vi "AlliGator Decay Analysis Actions.vi"(0 "AlliGator Q Elements in":T6[](array[typedef]), 1 "VI in":refnum<vi>, 2 "Script in":bool, 5 "AlliGator IV DVR in":refnum<data-value>, 7 "AlliGator Q Event in":T7=enum."GUI:Idle", 9 "Data":variant, 11 "error in (no error)":errorcluster, 12 "AlliGator Ctrl Refnums":T8) -> (3 "Script off":bool, 4 "AlliGator Q Elements out":T6[](array[typedef]), 6 "AlliGator IV DVR out":refnum<data-value>, 10 "[Notebook Message]":T1[](array[typedef]) {"Message Style"."Font Size" min=6.0 step=1.0}, 15 "error out":errorcluster)   [LabVIEW 2021, in "AlliGator Action Engine.lvlib"]
doc: "Processes AlliGator decay-related actions."
uses:
  AlliGator Action Engine.lvlib
  Internal Variables/AlliGator Internal Variables v2.ctl
  <vilib>/vision/Image Controls.llb/IMAQ Image.ctl
  Internal Variables/AlliGator Gate Image Set.ctl
  Files/AlliGator FLI Dataset Type.ctl
  Files/AlliGator Data Series Type.ctl
  Dual-Channel Datasets/AlliGator Dataset Channel.ctl
  Settings/AlliGator Gate Arithmetic.ctl
  Source Image/AlliGator Displayed Image.ctl
  Image/Named ROI Description.ctl
  Phasor Graph/AlliGator Decay Metadata v3.ctl
  Decay Analysis/Decay Preprocessing/AlliGator Decay Background Subtraction Info.ctl
  Decay Analysis/Decay Preprocessing/AlliGator Baseline Subtraction Method.ctl
  Graphs/XY Graph/XY Graph Plot Shift Parameters.ctl
  Graphs/XY Graph/XY Graph Plot Shift Method.ctl
  Decay Analysis/Decay Preprocessing/AlliGator Decay Extrapolation Parameters.ctl
  Phasor/Calibration Phasor (m, phi).ctl
  Phasor/Phasor Reference Series.ctl
  Phasor/Phasor Calibration Map v2.ctl
  Phasor/Phasor (g, s).ctl
  Phasor Graph/AlliGator Raw Phasor Plot Data v5.ctl
  Phasor/Phasor Standard Deviation Options.ctl
  Phasor Plot/AlliGator Phasor Multi-Harmonic Data.ctl
  Phasor/Phasor Harmonic Data.ctl
  Decay Fit Parameter Map/AlliGator Decay Fit Options & Parameters v4.ctl
  Fits/IRF(X)PSED/Decay Fit Options v4.ctl
  Fits/Decay Convolution/Decay Model.ctl
  Fits/Residual Type.ctl
  Fits/IRF(X)PSED/Fit Weights Type v2.ctl
  Fits/Non-linear Fitting Method v2.ctl
  Fits/Fit Calculation Method.ctl
  Fits/Non-linear Fitting Algorithm.ctl
  Decay Analysis/Decay Fit/AlliGator Decay Fit Parameter Constraints 2.ctl
  Fits/IRF(X)PSED/Decay Fit Parameters In List.ctl
  Fits/IRF(X)PSED/MLE Baseline Offset Type.ctl
  Decay Analysis/Decay Preprocessing/AlliGator Decay Preprocessing Parameters.ctl
  Fits/IRF(X)PSED/Decay Fit Parameters & Derived Quantities List v2.ctl
  Fits/IRF(X)PSED/Decay Fit Result Constraint.ctl
  Decay Fit Parameter Map/AlliGator Parameter Maps Data.ctl
  AlliGator Q Event.ctl
  GUI/AlliGator Ctrl Refnums.ctl
  GUI/AlliGator Other Ctrl Refnums.ctl
  GUI/AlliGator State Indicator.ctl
  GUI/AlliGator Main Window Tabs.ctl
  GUI/AlliGator Phasor Plot Ctrl Refnums.ctl
  GUI/AlliGator Phasor Graph Ctrl Refnums.ctl
  Phasor/Phasor Calibration Type.ctl
  GUI/AlliGator Dataset Ctrl Refnums.ctl
  GUI/AlliGator Registered Events Ctrl Refnums.ctl
  GUI/AlliGator Image Histogram Control Refnums.ctl
  Histograms/Linear Histogram Options.ctl
  Histograms/Histogram Bin Option.ctl
  Histograms/Histogram Bin Position.ctl
  Decay Fit Parameter Map/AlliGator Decay Fit Map Control Refnums.ctl
  Parameter Map/AlliGator Parameter Map Control Refnums.ctl
  AlliGator Q Element.ctl
  Notebook/Notebook Message Object.ctl
  Rich Text Box/Text Formatting.ctl
  Rich Text Box/Text Colors.ctl
  Rich Text Box/Text Style.ctl
  Rich Text Box/Text Alignment.ctl
  Rich Text Box/Text Format List.ctl
  Graphs/LabVIEW Plot Interpolation.ctl
  Graphs/Plot Point Style.ctl
  <vilib>/Utility/miscctls.llb/LVPoint32TypeDef.ctl
  Alligator Elements Order in Action Stack.ctl
  AlliGator State Indicators List.ctl
  Settings/AlliGator Settings List.ctl
  Graphs/XY Graph/XY Graph Selected Plot Info+Flag.ctl
  Graphs/XY Graph/XY Graph Refnum.ctl
  Fits/Square Pulse/Square Pulse Options.ctl
  Fits/Square Pulse/Square Pulse Levels Type.ctl
  Graphs/XY Graph/XY Graph Selected Plot Info.ctl
  Variant/Variant to Data/Variant to I32.vi
  AlliGator Add Single Action to Stack.vi
  AlliGator Add Action Array to Stack.vi
  Variant/Variant to Data/Variant to U32.vi
  Variant/Variant to Data/Variant to DBL.vi
  GUI/GUI.lvlib
  Decay Analysis/IRF/AlliGator IRF.lvlib
  Variant/Variant to Data/Variant to Data.lvlib
  GUI/AlliGator GUI.lvlib
  Decay Analysis/Decay Fit/AlliGator Decay Fit.lvlib
  Graphs/XY Graph/XY Graph Add-Ons.lvlib
  Decay Analysis/Decay Processing/AlliGator Decay Processing.lvlib
  Settings/AlliGator Settings.lvlib
  Internal Variables/AlliGator Internal Variables.lvlib
  Fits/Fits.lvlib
  Decay Analysis/Decay Preprocessing/AlliGator Decay Preprocessing.lvlib
  Graphs/Graphs.lvlib
  Decay Analysis/Global Decay Fit/AlliGator Global Decay Fit.lvlib
  Sound/Sound.lvlib
  Fits/Abort Fit Global.vi
  Intensity Corrections/AlliGator Intensity Corrections.lvlib
  Strings/Strings.lvlib
  Notebook/Notebook.lvlib
  Phasor/Phasor.lvlib
  Image/Image.lvlib
  Phasor Graph/AlliGator Phasor Graph.lvlib
  Files/AlliGator Files.lvlib
  Phasor Plot/AlliGator Phasor Plot.lvlib
  Source Image/AlliGator Source Image.lvlib
  Decay Fit Parameter Map/AlliGator Decay Fit Parameter Map.lvlib
  Rich Text Box/Rich Text Box.lvlib
  Dual-Channel Datasets/AlliGator Dual-Channel Datasets.lvlib
  Histograms/Histogram Window.lvlib
  Parameter Map/AlliGator Parameter Map.lvlib
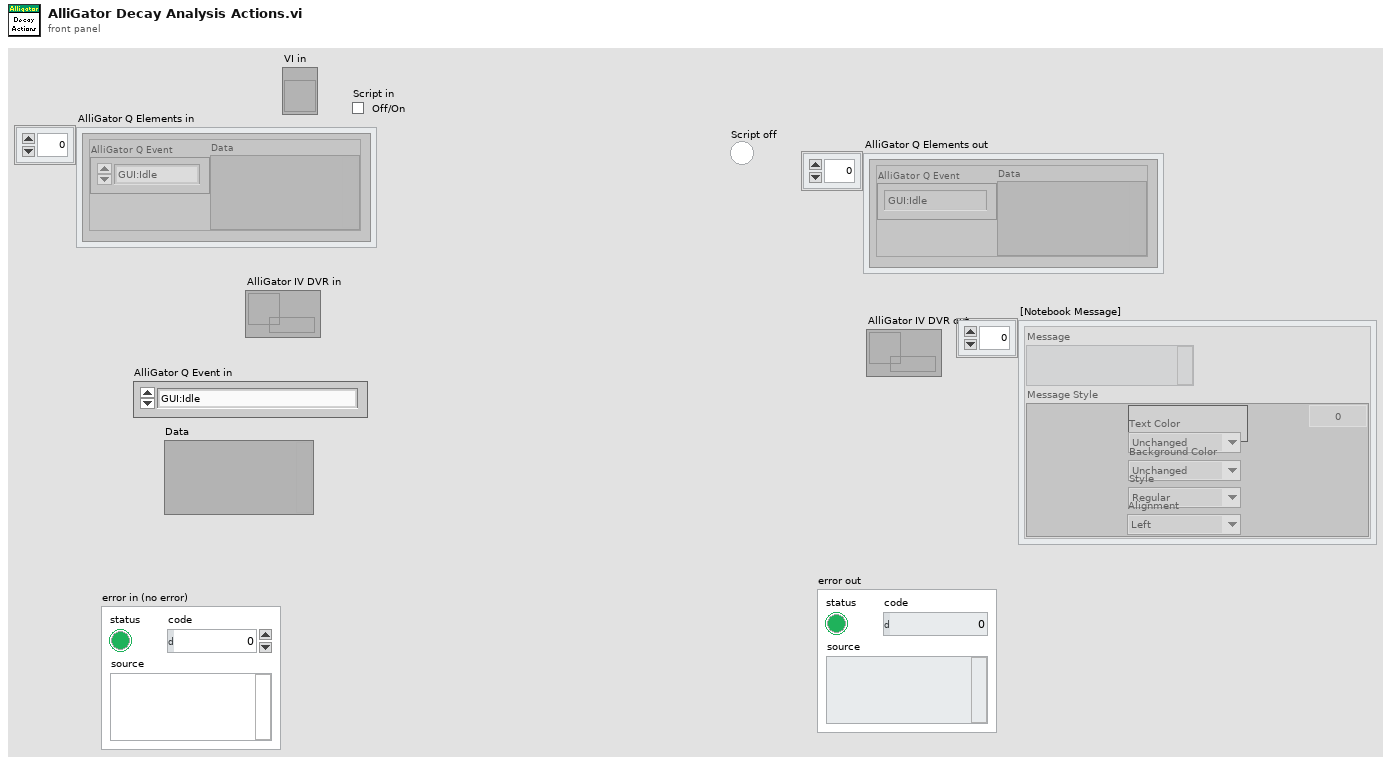
[diagram p1: front panel]
types:
  T1 = typedef "Notebook.lvlib/Notebook Message Object.ctl" = cluster{"Message":string, "Message Style":T2}
  T2 = typedef "Rich Text Box.lvlib/Text Formatting.ctl" = cluster{"Font":string, "Text Color":T3, "Background Color":T3, "Style":T4, "Font Size":dbl, "Alignment":T5}
  T3 = typedef "Rich Text Box.lvlib/Text Colors.ctl" = enum16{"Unchanged", "Black", "Blue", "Cyan", "Maroon", "Gray", "Violet", "Green", "Light Green", "Orange", "Yellow", "Magenta", "Red", "White"}
  T4 = typedef "Rich Text Box.lvlib/Text Style.ctl" = enum16{"Regular", "Bold", "Italic", "Underline", "Strikeout"}
  T5 = typedef "Rich Text Box.lvlib/Text Alignment.ctl" = enum16{"Left", "Right", "Center"}
  T6 = typedef "AlliGator Action Engine.lvlib/AlliGator Q Element.ctl" = cluster{"AlliGator Q Event":T7, "Data":variant}
  T7 = typedef "AlliGator Action Engine.lvlib/AlliGator Q Event.ctl" = enum16{"---- Files ----", "Files:Set Batch Export Files To Save", "Files:Set Dataset Loading & Pre-processing Options", "Files:Check #Frames in Dataset", "Files:Increment Frame Index", "Files:Open Mask Image", "Files:Open White Light Image", "Files:Open Single Dataset", "Files:New Folder of Folders Selected", "Files:Load File (all Types)_Scriptable", "Files:Move Flattened Series to Folders Series", "Files:Select Folder", "Files:Load FLI Dataset", "Files:Load Swiss SPAD 1 Dataset", "Files:Load Swiss SPAD 2 Dataset", "Files:Load .sdt FLI Dataset", "Files:Load .ptu FLI Dataset", "Files:Load .bin FLI Dataset", "Files:Load Single Gate Image Folder", "Files:Load I/m/phi Dataset (deprecated)", "Files:Load Single Image", "Files:Subtract Background File", "Files:Export FLI Dataset", "Files:Load HDF5 FLI Dataset", "Files:Set Destination File Path", "Files:Save Mask Image", "Files:Batch Conversion", "Files:New Folder Selected", "Files:Close FLI Dataset", "Files:Close FLI Dataset Series", "Files:Close White Light Image", "Files:Close Mask Image", "---- FLI Dataset ----", "FLI Dataset:Channel Arithmetic", "FLI Dataset:Export Average Lifetime Map as ASCII", "FLI Dataset:Export User-Defined Quantity Map as ASCII", "FLI Dataset:Python Function FLI Dataset Event", "FLI Dataset:ROI Analysis", "FLI Dataset:Tilted Logistic Square Gated IRF Characteristics Map", "FLI Dataset:Logistic Square Gated IRF Characteristics Map", "FLI Dataset:Square Gated IRF Characteristics Map", "FLI Dataset:Multi-ROI Single-Pixel Phasor Analysis", "FLI Dataset:Multi-ROI Single-Pixel NLSF Analysis", "FLI Dataset:All ROIs IRF Extraction", "FLI Dataset:All ROIs Decay Fit Non-Interactive (Fast + Individual IRF)", "FLI Dataset:All ROIs Phasor Analysis", "FLI Dataset:All ROIs Decay Fit", "FLI Dataset:Fluorescence Decay Statistics", "FLI Dataset:Update Decay Statistics Graph", "FLI Dataset:Get Decay from ROI", "FLI Dataset:All ROIs Average Lifetimes", "FLI Dataset:Save/Load Local IRFs", "FLI Dataset:Clear Local IRFs", "FLI Dataset:Phasor Calibration Maps (# Gates Series) Script", "FLI Dataset:Calibrated Phasor Map Series", "---- FLI Dataset Series ----", "FLI Dataset Series:Sum All Datasets in Series", "FLI Dataset Series:Add Dataset to Accumulated Dataset", "FLI Dataset Series:Display Accumulated Dataset", "FLI Dataset Series:Clear Dataset Series Sum", "FLI Dataset Series:Time-Series Analysis (NLSF)", "FLI Dataset Series:Time-Series Analysis (Phasor)", "---- Image ----", "Image:Update Image Profile Plots", "Image:Image Histogram Cursor Move", "Image:Image Histogram", "Image:Image Contrast", "Image:Set Image Histogram Cursor Move Flag", "Image:Clear Image Overlay", "Image:Use ROI as Search Area", "Image:Set ROI Diameter", "Image:Save Image Data as TIFF", "Image:Save Displayed Image with Overlay", "Image:Save Image Overlay Only", "Image:Save Image as Hot Pixel Mask", "Image:Change Source Image Color Palette", "Image:Copy Image to Clipboard", "Image:Source Image ROI Selection", "Image:Delete All ROIs", "Image:Delete All Unselected ROIs", "Image:Delete ROI", "Image:Merge All ROIs", "Image:Store ROI", "Image:Source Image ROI Storage", "Image:Export ROI Description to Notebook", "Image:Save ROI", "Image:Load ROI", "Image:Paste ROI Definition", "Image:Clear ROI", "Image:Identify ROIs in Mask Image", "Image:Create Complementary ROI", "Image:Create Contour ROI", "Image:Create ROI(s) from Pixels with Peak above Min_Scriptable", "Image:Create ROI(s) from Pixels with Intensity above Min_Scriptable", "Image:Compute ROI Statistics", "Image:Delete ROI(s) based on ROI Characteristics", "Image:Create ROI Grid", "Image:ROI to Individual Pixel ROIs", "Image:Python Function Source Image Event", "Image:Show Phasor Calibration Map ROI Centers", "Image:Convert ROI to Mask Image", "Image:Mouse Move", "Image:Mouse Up", "Image:Set Source Image Mouse Move Flag", "Image:Add Scale Bar Overlay", "Image:Delete Existing ROIs Option", "Image:Overlay ROI Median", "Image:Check Current ROI", "Image:Update True Pixel Value", "---- Decay ----", "Decay:Clear IRF/Reference Plot", "Decay:Add Decay to Graph", "Decay:Smoothen Plot", "Decay:Smoothen Plot Tail", "Decay:Average Selected Plots", "Decay:Extract IRF", "Decay:Optimal IRF Extraction", "Decay:Threshold IRF", "Decay:Fit to Model IRF", "Decay:Fit IRF to Square Gate", "Decay:Fit IRF to Logistic Square Gate", "Decay:Fit IRF to Tilted Logistic Square Gate", "Decay:Create Bounding Cursors Set", "Decay:Export Bounding Cursors Definition to Notebook", "Decay:Denoise Plot", "Decay:Compute Cumulative Function", "Decay:Use as Reference Decay", "Decay:Show Reference Decay/IRF", "Decay:Extrapolate Decay", "Decay:Create Head & Tail Bounding Cursors", "Decay:Store Cursor-defined Head & Tail Fractions", "Decay:Rebin Plot", "Decay:1-Normalize Decay", "Decay:[0-1]-Normalize Plot", "Decay:Straighten Decay", "Decay:Shift Decay", "Decay:Fold Decay", "Decay:Fit Decay", "Decay:Global Fit of Selected Decays", "Decay:Post Global Fit Script", "Decay:Add Global Fit Parameters to Graph", "Decay:Add Decay Parameter(s) to Plot (Graph)", "Decay:Export Decay to Phasor Graph", "Decay:Compute Average Lifetime", "Decay:Plot Convolution", "Decay:Graph Tip Strip Update", "---- Decay Statistics ----", "Decay Statistics:Tip Strip Update", "---- Intensity Time Trace ----", "Intensity Time Trace:Use File Timestamp", "Intensity Time Trace:Load Intensity Corrections File", "Intensity Time Trace:Clear Intensity Corrections File", "Intensity Time Trace:Tip Strip Update", "---- Phasor Plot ----", "Phasor Plot:Build Phasor Plot", "Phasor Plot:Change Phasor Plot Color Palette", "Phasor Plot:Adjust Phasor Plot Display Range", "Phasor Plot:Highlight Image ROI in Phasor Plot", "Phasor Plot:Save Phasor Plot Image with Overlay", "Phasor Plot:Export Complex Phasor Map", "Phasor Plot:Export Phasor Ratio Map", "Phasor Plot:Export Average Lifetime Map", "Phasor Plot:Compute Phase Lifetime Histogram", "Phasor Plot:Compute Phasor Ratio Histogram", "Phasor Plot:Compute Phase Lifetime vs Intensity Scatter Plot", "Phasor Plot:Weber 2-Component Decomposition", "Phasor Plot:Update Phasor Color Map Vertices", "Phasor Plot:Clear Phasor Overlay", "Phasor Plot:Use Segment Extremities as References", "Phasor Plot:Use UC/Segment Intersections as References", "Phasor Plot:Use UC/Principal Axis Intersections as References", "Phasor Plot:Use UC/Linear Fit Intersections as References", "Phasor Plot:Update Phasor Plot Reference", "Phasor Plot:Show Local Phasor Info in Phasor Plot", "Phasor Plot:Update Phasor Plot State", "Phasor Plot:Phasor Plot ROI Storage", "Phasor Plot:Phasor Plot ROI Selection", "Phasor Plot:Python Function Phasor Plot Event", "Phasor Plot:Overlay Phasor ROI, Ratio or Map in Source Image", "Phasor Plot:Compute Decay of Selected Phasors", "Phasor Plot:Phasor at Image Pixel", "Phasor Plot:Mouse Move", "Phasor Plot:Mouse Up", "Phasor Plot:Display Range Mouse Move", "Phasor Plot:Set Mouse Move Flag", "Phasor Plot:Update True Phasor Plot Value", "---- Phasor Graph ----", "Phasor Graph:Get Phasor Value", "Phasor Graph:Create New Phasor Plot Dialog", "Phasor Graph:Update Last Phasor Value", "Phasor Graph:Update Phasor (m, phi)", "Phasor Graph:Remove Single Phasor from Plot", "Phasor Graph:Add Single Phasor to Plot", "Phasor Graph:Remove Phasor Plot", "Phasor Graph:Remove Selected Phasor Plots", "Phasor Graph:Clear Phasor Data", "Phasor Graph:Clear Phasor Graph", "Phasor Graph:Cursor Move", "Phasor Graph:Draw Cursor Connecting Line", "Phasor Graph:Clear Cursor Connecting Line", "Phasor Graph:Find UC Intersection", "Phasor Graph:Use UC/Cursor-Defined Line Intersections", "Phasor Graph:Use Selected Plots Fitted Line/UC Intersections", "Phasor Graph:Use Selected Plots Principal Axis/UC Intersections", "Phasor Graph:Show Single Phasor", "Phasor Graph:Save Single Phasor Plot", "Phasor Graph:Save All Phasor Plots", "Phasor Graph:Load Phasor Plot(s)", "Phasor Graph:Phasor Multiplication", "Phasor Graph:Compute Average Phasor", "Phasor Graph:Compute Multiple Average Phasors (Selected Plots)", "Phasor Graph:Export Single Phasor Plot Phase Lifetimes", "Phasor Graph:Parameter 2 vs Parameter 1 Scatter Plot", "Phasor Graph:Use Cursor n Location", "Phasor Graph:Set Reference n to Current Phase Lifetime Value", "Phasor Graph:Set Reference n to Lifetime Value", "Phasor Graph:Set Cursor n Location", "Phasor Graph:Save Phasor Graph Image", "Phasor Graph:Update SEPL Plot", "Phasor Graph:Export Single Phasor Plot Data", "Phasor Graph:Export Selected Phasor Plots Data", "Phasor Graph:Python Function Phasor Graph Event", "Phasor Graph:Tip Strip Update", "---- Calibration ----", "Calibration:Set Calibration Type", "Calibration:Load/Save Phasor Calibration", "Calibration:Load/Save Phasor Calibration Series", "Calibration:Load/Save Phasor Calibration Map", "Calibration:Use as Calibration", "Calibration:Compute Optimal Calibration from Phasor References", "Calibration:Clear Phasor Calibration", "Calibration:Single Phasor Calibration Information", "Calibration:Use as Calibration Series", "Calibration:Use as Calibration Map", "Calibration:Clear Calibration Series", "Calibration:Phasor Calibration Series Information", "Calibration:Clear Calibration Map", "Calibration:Phasor Calibration Map Information", "Calibration:Apply Phasor Calibration", "Calibration:Update Single Plot Calibration", "Calibration:Update Multiple Plots Calibration", "Calibration:Clear Single Plot Calibration", "Calibration:Clear All Plots Calibrations", "Calibration:Clear Plot(s) Calibration(s)?", "---- Phasor Ratio ----", "Phasor Ratio:Clear Reference n", "Phasor Ratio:Toggle Selected Plot(s)  Lock to Reference 1", "Phasor Ratio:Use as Reference n", "Phasor Ratio:Send Reference n to Notebook", "Phasor Ratio:Toggle Selected Plot(s)  Lock to Reference 2", "Phasor Ratio:Compute Phasor Ratio at Mouse Location", "Phasor Ratio:Compute Phasor Plot's Average Phasor Ratio", "Phasor Ratio:Compute Time-Series Phasor Ratios", "Phasor Ratio:Fit Line to Phasor Ratio Plot", "Phasor Ratio:Save References", "Phasor Ratio:Load References", "Phasor Ratio:Update Phasor Reference 1", "Phasor Ratio:Update Phasor Reference 2", "Phasor Ratio:Move Cursor n to Reference n", "Phasor Ratio:Use as Phasor Reference 1 Lifetime", "Phasor Ratio:Use as Phasor Reference 2 Lifetime", "Phasor Ratio:Export Phasor Ratio Map as ASCII", "Phasor Ratio:Tip Strip Update", "---- Lifetime & Other Parameters Graph ----", "Lifetime:Compute Sliced Mean, SDV and CV Plots", "Lifetime:Plot Decay Shifts", "Lifetime:Plot Histogram", "---- Decay Fit Parameter Map ----", "Decay Fit Parameter Map:Export ROI NLSF Data as ASCII", "Decay Fit Parameter Map:Set Decay Fit Parameter Map Selection", "Decay Fit Parameter Map:Build Decay Fit Parameter Map", "Decay Fit Parameter Map:Change Decay Fit Parameter Map Color Palette", "Decay Fit Parameter Map:Export Decay Fit Parameter Map Data as ASCII", "Decay Fit Parameter Map:Export All Decay Fit Parameter Maps Data as ASCII", "Decay Fit Parameter Map:Selected Parameter Scatterplot", "Decay Fit Parameter Map:Parameter 2 vs Parameter 1 Scatterplot", "Decay Fit Parameter Map:Save Decay Fit Parameter Map Image", "Decay Fit Parameter Map:Save-Load IRFs & Fit Data", "Decay Fit Parameter Map:Update Local Decay Plots", "Decay Fit Parameter Map:Python Function Decay Fit Parameters Map Event", "Decay Fit Parameter Map:Overlay Decay Fit Parameter Map in Source Image", "Decay Fit Parameter Map:Selected Parameter vs Intensity Scatterplot", "Decay Fit Parameter Map:Mouse Up", "Decay Fit Parameter Map:Mouse Move", "Decay Fit Parameter Map:Display Range Mouse Move", "Decay Fit Parameter Map:Change Map Resolution", "Decay Fit Parameter Map:Variance Significance Maps", "Decay Fit Parameter Map:Fit Result Constraints Window", "---- Parameter Map ----", "Parameter Map:Export ROI Parameters Data as ASCII", "Parameter Map:Add Parameter Map Set", "Parameter Map:Delete Parameter Map Set", "Parameter Map:Update Parameter List", "Parameter Map:Build Parameter Map", "Parameter Map:Change Parameter Map Color Palette", "Parameter Map:Export Parameter Map Data as ASCII", "Parameter Map:Export All Parameter Maps Data as ASCII", "Parameter Map:Selected Parameter Scatterplot", "Parameter Map:Parameter 2 vs Parameter 1 Scatterplot", "Parameter Map:Selected Parameter vs Intensity Scatterplot", "Parameter Map:Save Parameter Map Image", "Parameter Map:Save-Load IRFs & Parameter Maps (TODO)", "Parameter Map:Set Parameter Map Selection", "Parameter Map:Python Function Parameter Map Event", "Parameter Map:Overlay Parameter Map in Source Image", "Parameter Map:Update Local Decay Plots", "Parameter Map:Mouse Up", "Parameter Map:Mouse Move", "Parameter Map:Display Range Mouse Move", "---- Generic Graph ----", "Generic Graph:Generic XY Graph Event", "Generic Graph:Python Function XY Graph Event", "Generic Graph:New Plot", "Generic Graph:Save Plot", "Generic Graph:XY Plot Histogram", "Generic Graph:Set XY Graph Plot Name", "Generic Graph:Set Last Cursor Style", "Generic Graph:Tip Strip Update", "---- GUI ----", "GUI:Start Script", "GUI:Type of Displayed Image Changed", "GUI:Gate Image Slide Changed", "GUI:Show Busy Icon", "GUI:Show Busy Icon & Abort Button", "GUI:Hide Busy Icon", "GUI:Hide Busy Icon & Abort Button", "GUI:Abort", "GUI:End Script", "GUI:Start Timing", "GUI:End Timing", "GUI:Set State Indicator", "GUI:Send Parameters JSON Strings to Clipboard", "GUI:Set Gate Step", "GUI:Idle", "GUI:Initialization", "GUI:Quit", "GUI:Increment Dataset Index", "GUI:Set Dataset Index to -1", "GUI:Time Series Slider Moved", "GUI:Time Series Slider Changed", "GUI:Toggle Playback or Loop", "GUI:Playback Script", "GUI:Set Phasor Frequency", "GUI:Open Window", "GUI:Start Test Script", "GUI:End Test Script", "GUI:Set Verbose Mode", "GUI:Set Verbose Settings Mode", "DEBUG"}
  T8 = typedef "AlliGator GUI.lvlib/AlliGator Ctrl Refnums.ctl" = cluster{"Other AlliGator Ctrl Refnums":T9, "Phasor Plot Ctrl Refnums":T10, "Phasor Graph Ctrl Refnums":T11, "Dataset Control Refnums":T12, "Registered Events Ctrl Refnums":T13, "Image Histogram Ctrl Refnums":T14, "Decay Fit Map Ctrl Refnums":T15, "Parameter Map Ctrl Refnums":T16}
  T9 = typedef "AlliGator GUI.lvlib/AlliGator Other Ctrl Refnums.ctl" = cluster{"State Indicators":refnum<vi>, " Progress Bar":refnum<vi>, "Decay Graph Active":refnum<vi>, "Decay Statistics Bin":refnum<vi>, "Time Step":refnum<vi>, "Use File Timestamp":refnum<vi>, "Tab Control":refnum<vi>, "CPU":refnum<vi>, "Abort Fit":refnum<vi>, "Dataset File/Folder Path":refnum<vi>, "Abort ROI Creation":refnum<vi>, "Event LED":refnum<vi>, "Dataset File/Folder Path 2":refnum<vi>, "Dataset File/Folder Path 3":refnum<vi>, "Dataset File/Folder Path 4":refnum<vi>, "Dataset File/Folder Path 5":refnum<vi>, "Dataset File/Folder Path 6":refnum<vi>, "Dataset File/Folder Path 7":refnum<vi>, "Dataset File/Folder Path 8":refnum<vi>, "Dataset File/Folder Path 9":refnum<vi>, "Dataset File/Folder Path 10":refnum<vi>, "Dataset File/Folder Path 11":refnum<vi>}
  T10 = typedef "AlliGator GUI.lvlib/AlliGator Phasor Plot Ctrl Refnums.ctl" = cluster{"Phasor Ratio":refnum<vi>, "Modulus Lifetime":refnum<vi>, "Phasor at cursor (m, phi)":refnum<vi>, "Phase Lifetime":refnum<vi>, "Phasor at cursor (g, s)":refnum<vi>, "Phasor Plor Average Lifetime":refnum<vi>, "Phasor Plot Active":refnum<vi>, "Save Phasor Plot":refnum<vi>, "Image Overlay Color":refnum<vi>, "Phasor Plot Color Scale":refnum<vi>, "Reference 1 Button":refnum<vi>, "Reference 2 Button":refnum<vi>, "True Phasor Plot Value":refnum<vi>}
  T11 = typedef "AlliGator GUI.lvlib/AlliGator Phasor Graph Ctrl Refnums.ctl" = cluster{"Phasor Ratio":refnum<vi>, "Modulus Lifetime":refnum<vi>, "Phasor at cursor (m, phi)":refnum<vi>, "Phase Lifetime":refnum<vi>, "Phasor at cursor (g, s)":refnum<vi>, "Phasor Graph Average Lifetime":refnum<vi>, "Phasor Graph Active":refnum<vi>, "Save Phasor Graph":refnum<vi>, "Phasor Frame Slide":refnum<vi>, "Single Step Phasor":refnum<vi>, "Calibration Type":refnum<vi>, "Show Line":refnum<vi>, "Phase Lifetime 1":refnum<vi>, "Phase Lifetime 2":refnum<vi>, "Phasor Graph Frequency":refnum<vi>, "Phasor Reference 1 Control":refnum<vi>, "Phasor Reference 2 Control":refnum<vi>, "Calibration Lifetime":refnum<vi>, "Phase Lifetime SDV":refnum<vi>, "Average Lifetime SDV":refnum<vi>, "Phasor Ratio SDV":refnum<vi>, "Modulus Lifetime SDV":refnum<vi>}
  T12 = typedef "AlliGator GUI.lvlib/AlliGator Dataset Ctrl Refnums.ctl" = cluster{"Current Data":refnum<vi>, "Gate Image Slide":refnum<vi>, "Time Point Slide":refnum<vi>, "Current Time Stamp":refnum<vi>, "Save Image":refnum<vi>, "Displayed Image":refnum<vi>, "Overlay Mode":refnum<vi>, "Phasor Overlay Color":refnum<vi>, "Image Color Scale":refnum<vi>, "Use ROI as Search Area":refnum<vi>, "Source Image ROI Color":refnum<vi>, "True Pixel Value":refnum<vi>}
  T13 = typedef "AlliGator GUI.lvlib/AlliGator Registered Events Ctrl Refnums.ctl" = cluster{"Time Point Slider":refnum<vi>, "Phasor Plot Display Range":refnum<vi>, "Decay Graph":refnum<vi>, "Decay Statistics Graph":refnum<vi>, "Intensity Time Trace":refnum<vi>, "Phasor Graph":refnum<vi>, "Phasor Ratio Graph":refnum<vi>, "Lifetime Graph":refnum<vi>, "Phasor Plot Display":refnum<vi>, "Source Image Display":refnum<vi>, "Decay Fit Parameter Map Display Range":refnum<vi>, "Decay Fit Parameter Map Display":refnum<vi>, "Parameter Map Display Range":refnum<vi>, "Parameter Map Display":refnum<vi>, "Phasor Plot Display Range":refnum<vi>}
  T14 = typedef "AlliGator GUI.lvlib/AlliGator Image Histogram Control Refnums.ctl" = cluster{"Image Histogram":refnum<vi>, "Image Histogram Options":refnum<vi>, "Image Histogram Active":refnum<vi>, "Image Histogram Upper Percentile":refnum<vi>, "Image Histogram Lower Percentile":refnum<vi>, "Auto-Adjust Contrast":refnum<vi>}
  T15 = typedef "AlliGator Decay Fit Parameter Map.lvlib/AlliGator Decay Fit Map Control Refnums.ctl" = cluster{"Decay Fit Parameter Map Color Scale":refnum<vi>, "Decay Fit Parameter":refnum<vi>, "Max Parameter":refnum<vi>, "Min Parameter":refnum<vi>, "Decay Fit Parameter Map Display":refnum<vi>, "Decay Fit Parameter Map Display Range":refnum<vi>, "Decay Parameter Map X":refnum<vi>, "Decay Parameter Map Y":refnum<vi>, "Decay Parameter Map Value":refnum<vi>}
  T16 = typedef "AlliGator Parameter Map.lvlib/AlliGator Parameter Map Control Refnums.ctl" = cluster{"Parameter Map Color Scale":refnum<vi>, "Map Parameter":refnum<vi>, "Max Parameter":refnum<vi>, "Min Parameter":refnum<vi>, "Parameter Map Display":refnum<vi>, "Parameter Map Display Range":refnum<vi>, "Parameter Map Set":refnum<vi>, "Parameter Map X":refnum<vi>, "Parameter Map Y":refnum<vi>, "Parameter Map Value":refnum<vi>}
  T17 = typedef "Notebook.lvlib/Text Format List.ctl" = enum16{"Message", "Result", "Error", "Setting", "Verbose", "Warning"}
  T18 = typedef "Graphs.lvlib/Plot Point Style.ctl" = enum16{"not defined", "None", "Empty Circle", "Filled Circle", "Thick Circle", "Dotted Circle", "Empty Square", "Filled Square", "Thick Square", "Dotted Square", "Small Filled Square", "Dot", "Cross", "Tiny Cross", "Large X", "Small x", "Diamond", "Small Empty Square"}
  T19 = typedef "Graphs.lvlib/LabVIEW Plot Interpolation.ctl" = enum16{"Point (.)", "Stepwise Right (--.)", "Line + Point (\\. /)", "Stepwise Left (.--)", "Stepwise Centered (-.-)", "Stepwise Vertical (|.|)", "Line (-)", "Use Previous Plot's Style"}
  T20 = typedef "AlliGator Action Engine.lvlib/Alligator Elements Order in Action Stack.ctl" = enum16{"Enqueue 2 AFTER 1", "Enqueue 2 BEFORE 1"}
  T21 = typedef "AlliGator Action Engine.lvlib/AlliGator State Indicators List.ctl" = enum16{"Phasor Calibration Defined", "Phasor Calibration Series Defined", "Phasor Calibration Map Defined", "Phasor Reference 1 Defined", "Phasor Reference 2 Defined", "Lifetime Reference 1 Defined", "Lifetime Reference 2 Defined", "Phasor Calibration Used", "Phasor Calibration Series Used", "Phasor Calibration Map Used", "Dataset Update Needed", "Phasor Plot Update Needed", "Reference/IRF Defined", "Individual IRFs Defined"}
  T22 = typedef "AlliGator Settings.lvlib/AlliGator Settings List.ctl" = enum16{"GUI:Visible Settings Tab", "GUI:Last Run Version", "Source Image:Use Image Histogram for Contrast", "Source Image:Low Count Pixels Rejection Options", "Source Image:High Count Pixels Rejection Options", "Source Image:Use Image Brightness", "Source Image:Blend Overlay with Image Background", "Source Image:Use Fixed ROI Diameter", "Source Image:ROI Diameter", "Source Image:ROI Center Color", "Source Image:Peak Threshold", "Source Image:Intensity Threshold", "Source Image:Image Binning Options", "Source Image:Image Smoothing Options", "Source Image:Image Histogram Active", "Source Image:Invert Binary Mask", "Source Image:Hot Pixel Removal", "Source Image:Overlay Analyzed ROI Center", "Source Image:Auto-Adjust Contrast", "Source Image:Histogram Lower Percentile", "Source Image:Histogram Upper Percentile", "Source Image:Save Source Image", "Source Image:Scale Bar Options", "Source Image:Image Resolution (Pixel Size)", "Source Image:Flatfield Correction", "Source Image:Show Dead Left Columns Correction", "Source Image:Dead Left Columns Correction", "Source Image:Image Pre-Processing Operations Order", "Source Image:Overlay ROI Median", "Source Image:Median Overlay Color", "Data Information:Gate Width", "Data Information:Nanotime Gate Separation", "Data Information:Macrotime Gate Separation", "Data Information:Gate Step", "Data Information:# Gates", "Data Information:Gate Image Exposure", "Data Information:Gate Image Integration", "Data Information:Gates to Skip", "Data Information:Gates to Keep", "Data Information:Define Gates to", "Data Information:Channel Name", "Data Information:Available Channel Names", "Data Information:Channel Arithmetic", "Data Information:Background File Subtraction", "Data Information:Background File", "Data Information:Background Scaling Factor", "Data Information:Background Pile-up Correction", "Data Information:Background Pixel Well Capacity", "Data Information:Laser Period", "Data Information:SYNC Period", "Data Information:Pile-up Correction", "Data Information:Pixel Well Capacity", "Data Information:Dataset Scaling Factor", "Fluorescence Decay_Decay Pre-Processing:Reverse Gates", "Fluorescence Decay_Decay Pre-Processing:Verbose Decay Pre-Processing", "Fluorescence Decay_Decay Pre-Processing:Use Decay Pre-Processing", "Fluorescence Decay_Decay Pre-Processing:Background Subtraction", "Fluorescence Decay_Decay Pre-Processing:Background Definition Range", "Fluorescence Decay_Decay Pre-Processing:Baseline Subtraction Method", "Fluorescence Decay_Decay Pre-Processing:Decay Pre-Processing Operations Order", "Fluorescence Decay_Decay Pre-Processing:Smoothing Parameter", "Fluorescence Decay_Decay Pre-Processing:Shift Decay", "Fluorescence Decay_Decay Pre-Processing:Decay Shift Parameters", "Fluorescence Decay_Decay Pre-Processing:Fold Decay", "Fluorescence Decay_Decay Pre-Processing:# Folds", "Fluorescence Decay_Decay Pre-Processing:1-Normalize Decay", "Fluorescence Decay_Decay Pre-Processing:[0-1]-Normalize Decay", "Fluorescence Decay_Decay Pre-Processing:Smoothen Decay", "Fluorescence Decay_Decay Pre-Processing:Extrapolate Decay", "Fluorescence Decay_Decay Pre-Processing:Use Periodicity", "Fluorescence Decay_Decay Pre-Processing:Use Cursors", "Fluorescence Decay_Decay Pre-Processing:Tail Fraction", "Fluorescence Decay_Decay Pre-Processing:Head Fraction", "Fluorescence Decay_Decay Pre-Processing:Additional Points", "Fluorescence Decay_Decay Pre-Processing:Straighten Decay", "Fluorescence Decay_Decay Pre-Processing:Constant Background", "Fluorescence Decay_Decay Pre-Processing:Pixel-Normalize Decay", "Fluorescence Decay_Advanced Analysis:Extract IRF instead of Decay", "Fluorescence Decay_Advanced Analysis:IRF Extraction Options", "Fluorescence Decay_Advanced Analysis:IRF Optimization Options", "Fluorescence Decay_Advanced Analysis:Square Pulse Options", "Fluorescence Decay_Advanced Analysis:IRF Order", "Fluorescence Decay_Advanced Analysis:IRF Time Constants", "Fluorescence Decay_Advanced Analysis:Wavelet Analysis Options", "Fluorescence Decay_Advanced Analysis:Average Lifetime Options", "Fluorescence Decay_Fit Options:Fit Options", "Fluorescence Decay_Fit Options:Use Legacy Fitting Approach", "Fluorescence Decay_Fit Options:Use Data Information Laser Period", "Fluorescence Decay_Fit Parameters:Displayed Fit Parameters", "Fluorescence Decay_Fit Parameters:Fit Parameter Constraints", "Fluorescence Decay_Fit Parameters:Export Tabulated Results", "Fluorescence Decay_Fit Parameters:MLE Baseline Offset Type", "Fluorescence Decay_Fit Parameters:MLE Baseline Offset", "Fluorescence Decay_Fit Parameters:Guess Parameter Names", "Fluorescence Decay_Fit Parameters:Guess Parameter Values", "Fluorescence Decay_Fit Parameters:Guess Parameters Options", "Fluorescence Decay_Fit Parameters:Optimal Offset Selection Criterion", "Fluorescence Decay_Styles:Show Last Decay Only", "Fluorescence Decay_Styles:Decay Graph Color Array", "Fluorescence Decay:Decay Graph Active", "Fluorescence Decay Statistics:Min Peak Value", "Fluorescence Decay Statistics:Reject Low Decay Peak Pixels", "Fluorescence Decay Statistics:Reject High Decay Peak Pixels", "Fluorescence Decay Statistics:Max Peak Value", "Time Traces:Use File Timestamp", "Time Traces:Time Step", "Time Traces:Use Intensity Correction File", "Time Traces:Intensity Correction File", "Phasor Plot:Phasor Plot Smoothing Options", "Phasor Plot:Phasor Plot Size", "Phasor Plot:Phasor Plot Graphics Options", "Phasor Plot:Cumulative Phasor Plot", "Phasor Plot:Use Phasor Brightness", "Phasor Plot:Blend Overlay with Phasor Background", "Phasor Plot:Save Phasor Plot", "Phasor Plot:Show References", "Phasor Plot:Phasor Ratio Decay Range", "Phasor Plot:Exponential Fading", "Phasor Plot:Phasor Ratio Reference Colors", "Phasor Plot:Reference Radius", "Phasor Plot:Show Color Map Vertices", "Phasor Plot:Phasor Plot Active", "Phasor Plot:Phasor Ratio Color Map Type", "Phasor Plot:Phasor Ratio Color Map", "Phasor Plot:Phasor Ratio Display Range", "Phasor Plot:Selected Image ROI(s)", "Phasor Plot:All Image ROIs", "Phasor Plot:Selected Phasor Plot ROI(s)", "Phasor Plot:All Phasor Plot ROIs", "Phasor Plot:Phasor Ratio Color-Coded Quantity", "Phasor Plot:Store Phasor Harmonics", "Phasor Plot:Draw Reference Segment", "Phasor Plot:User-Defined Quantity", "Phasor Plot:Color Scale High Color", "Phasor Plot:Color Scale Low Color", "Phasor Plot:Intensity-weighted Phasor Plot", "Phasor Graph:Phasor Frequency", "Phasor Graph:Phasor Ratio Type", "Phasor Graph:Pixel-level Phasor Computation", "Phasor Graph:Save Phasor Graph", "Phasor Graph:Phasor Graph Active", "Phasor Graph:Phasor SDV Options", "Phasor Graph:Intensity-weighted Phasor Graph", "Phasor Graph:Define Shortest Lifetime as", "Phasor Calibration:Use Backup Calibration if needed", "Phasor Calibration:Backup Calibration Type", "Phasor Calibration:Calibration Type", "Phasor Calibration:Calibration Lifetime", "Phasor Calibration:Calibration Map Algorithm", "Single-Exponential Phasor Locus (SEPL):Gate Parameters", "Single-Exponential Phasor Locus (SEPL):User-defined Gate", "Single-Exponential Phasor Locus (SEPL):User-defined IRF", "Single-Exponential Phasor Locus (SEPL):Phasor Parameters", "Single-Exponential Phasor Locus (SEPL):Decay & IRF Parameters", "Single-Exponential Phasor Locus (SEPL):Display Parameters", "Lifetime Analysis:Decay Analysis Parameters", "Lifetime Analysis:Lifetime Map Active", "Plugins:Python Settings", "Miscellaneous:Verbose Mode", "Miscellaneous:Beep after Script", "Miscellaneous:Saved Image File Format", "Miscellaneous:Exported Gate Image Settings", "Miscellaneous:Include Loading in Timing", "Miscellaneous:Verbose Settings Mode", "Miscellaneous:Histogram Options", "Miscellaneous:Beep on Error", "Miscellaneous:# Logical Processors Used", "Miscellaneous:ROI Description Max Characters", "Miscellaneous:Verbose Error Mode", "Miscellaneous:Transparent Mask Color"}
  T23 = typedef "XY Graph Add-Ons.lvlib/XY Graph Selected Plot Info+Flag.ctl" = cluster{"Multiplot XY Graph":T24, "Mouse Coordinates":T25, "Plot Index":i32, "Flag":bool}
  T24 = typedef "XY Graph Add-Ons.lvlib/XY Graph Refnum.ctl" = refnum<vi>
  T25 = typedef "LVPoint32TypeDef.ctl" = cluster{"Horizontal":i32, "Vertical":i32}
  T26 = typedef "Fits.lvlib/Square Pulse Options.ctl" = cluster{"Method":T27, "# Bins":i32, "Threshold %":dbl, "Center on Midpoint":bool, "Smoothen Plot":bool}
  T27 = typedef "Fits.lvlib/Square Pulse Levels Type.ctl" = enum16{"Mode", "Mean"}
  T28 = typedef "XY Graph Add-Ons.lvlib/XY Graph Selected Plot Info.ctl" = cluster{"Multiplot XY Graph":T24, "Mouse Coordinates":T25, "Plot Index":i32}
  T29 = typedef "AlliGator Decay Fit.lvlib/AlliGator Decay Fit Output Options.ctl" = cluster{"Fit Model":T30, "Decay Fit Parameter Array":T31[]}
  T30 = typedef "Fits.lvlib/Decay Model.ctl" = enum16{"1-Exponential", "2-Exponentials"}
  T31 = typedef "Fits.lvlib/Decay Fit Parameters & Derived Quantities List v2.ctl" = enum16{"Offset", "Baseline", "A_1", "tau_1", "A_2", "tau_2", "<tau>_a", "f1_a", "f2_a", "<tau>_i", "f1_i", "f2_i", "-", "R^2", "Chi^2"}
  T32 = cluster{"CtlRef":refnum<vi>, "Coords":T25, "Plot ID":i32}
  T33 = typedef "Math.lvlib/Wavelet Analysis Options.ctl" = cluster{"Wavelet":enum16{"db02", "db03", "db04", "db05", "db06", "db07", "db08", "db09", "db10", "db11", "db12", "db13", "db14", "Haar", "bior1_3", "bior1_5", "bior2_2", "bior2_4", "bior2_6", "bior2_8", "bior3_1", "bior3_3", "bior3_5", "bior3_7", "bior3_9", "bior4_4 (FBI)", "bior5_5", "bior6_8", "coif1", "coif2", "coif3", "coif4", "coif5", "sym2", "sym3", "sym4", "sym5", "sym6", "sym7", "sym8"}, "Option for Approximate Coefficients":enum16{"None", "Threshold", "Detrend"}, "# Levels":i32, "Threshold Settings":cluster{"Thresholding Rule":enum16{"SURE", "Hybrid", "Universal", "Minimax"}, "Rescaling Method":enum16{"One", "Single level", "Multiple levels"}, "Soft Threshold?":bool}, "Wavelet Transform Type":enum16{"Discrete", "Undecimated"}}
  T34 = typedef "ROI Descriptor" = cluster{"Global Rectangle":i32[], "Contours":cluster{"ID":enum32{"External", "Internal"}, "Type":u32, "Coordinates":i32[]}[]}
  T35 = typedef "XY Graph Add-Ons.lvlib/XY Graph Plot Data.ctl" = cluster{"X Array":dbl[], "Y Array":dbl[]}
  T36 = typedef "AlliGator Decay Fit Parameter Map.lvlib/AlliGator Decay Fit Options & Parameters v4.ctl" = cluster{"SYNC Period":dbl[unit], "Fit Options":T37, "Fit Parameter Constraints":T43[], "MLE Baseline Offset":dbl, "MLE Baseline Offset Type":T45}
  T37 = typedef "Fits.lvlib/Decay Fit Options v4.ctl" = cluster{"Show Fit Residuals":bool, "Fit Model":T30, "Residual Type":T38, "Max Decay Percentile":dbl, "Min Decay Percentile":dbl, "Show Full Decay":bool, "Weights":T39, "Fitting Method":T40, "Compute Parameter Uncertainties":bool, "Periodic Boundaries":bool, "Model Calculation":T41, "Period":dbl[unit], "Termination Criteria":cluster{"Max Iterations":i32, "Max Function Calls":i32, "Max Time":dbl[unit], "Function Tolerance":dbl, "Parameter Tolerance":dbl, "Gradient Tolerance":dbl, "Min Lambda":dbl, "Max Lambda":dbl, "Initial Tick Count":u32}, "Offset Resolution":dbl[unit], "Use Local IRF":bool, "Fitting Algorithm":T42, "Show Confidence Interval ":bool, "Confidence Level":dbl}
  T38 = typedef "Fits.lvlib/Residual Type.ctl" = enum16{"Standard", "Normalized", "Reduced"}
  T39 = typedef "Fits.lvlib/Fit Weights Type v2.ctl" = enum16{"Unweighted", "1/Variance (Neyman)", "1/Variance (Pearson)", "Best of All"}
  T40 = typedef "Fits.lvlib/Non-linear Fitting Method v2.ctl" = enum16{"Least Square", "Least Absolute Residual", "Bisquare", "MLE", "-", "Best of All"}
  T41 = typedef "Fits.lvlib/Fit Calculation Method.ctl" = enum16{"Simulation", "Convolution", "Integration"}
  T42 = typedef "Fits.lvlib/Non-linear Fitting Algorithm.ctl" = enum16{"Levenberg-Marquardt", "Trust-Region Dogleg"}
  T43 = typedef "AlliGator Decay Fit.lvlib/AlliGator Decay Fit Parameter Constraints 2.ctl" = cluster{"Fit Parameter":T44, "Min Value":dbl, "Max Value":dbl, "Global":bool, "Used":bool}
  T44 = typedef "Fits.lvlib/Decay Fit Parameters In List.ctl" = enum16{"Offset", "Baseline", "A_1", "tau_1", "A_2", "tau_2"}
  T45 = typedef "Fits.lvlib/MLE Baseline Offset Type.ctl" = enum32{"Absolute", "Percentage"}
  T46 = cluster{"t Array":dbl[], "Amplitude Array":dbl[]}
  T47 = typedef "XY Graph Add-Ons.lvlib/XY Graph Plot Shift Parameters.ctl" = cluster{"Type":T48, "Shift":dbl[unit], "Threshold":dbl, "Rotate":bool}
  T48 = typedef "XY Graph Add-Ons.lvlib/XY Graph Plot Shift Method.ctl" = enum16{"Default", "CFD", "Threshold", "Cross-Correlation"}
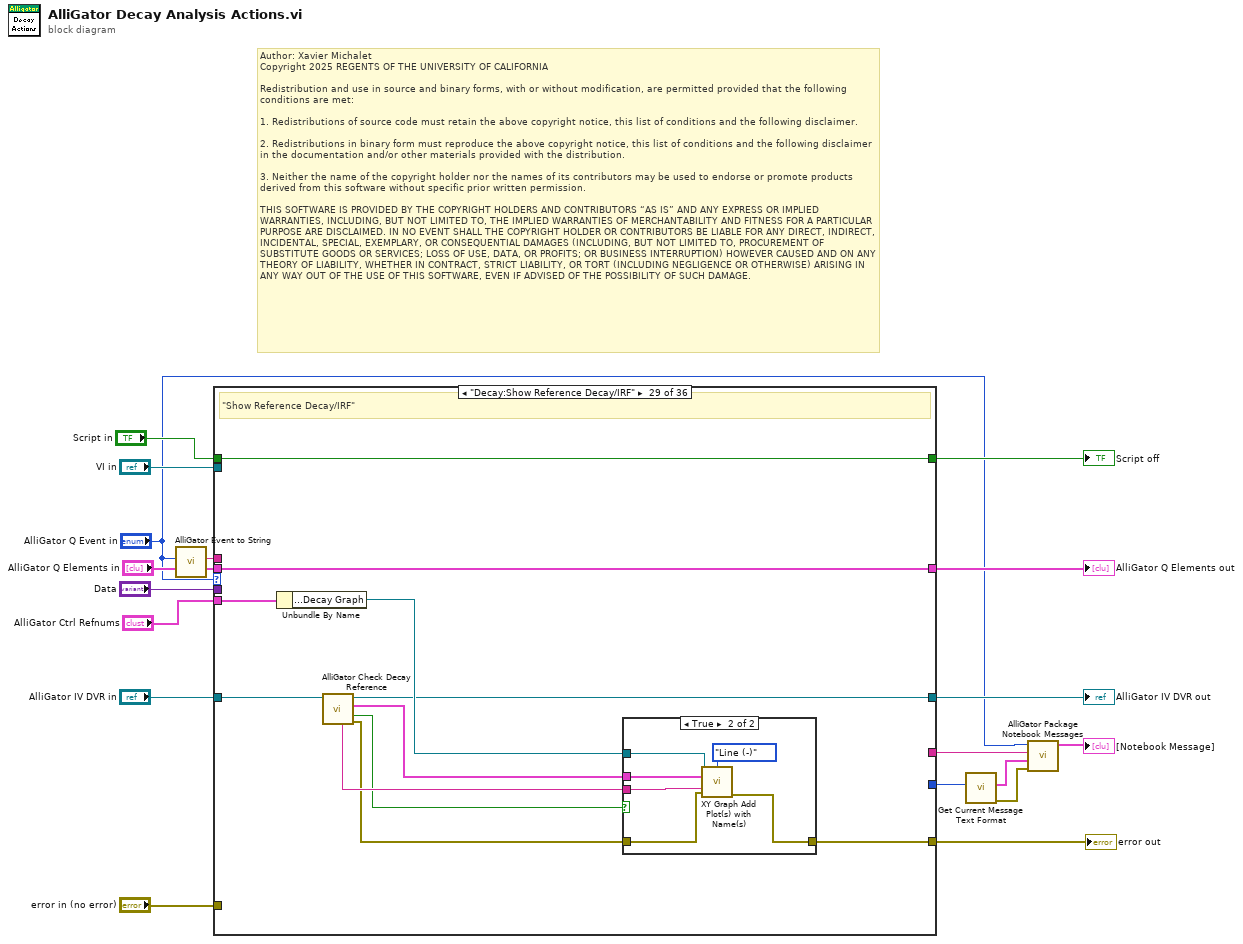
[diagram p0: block diagram]
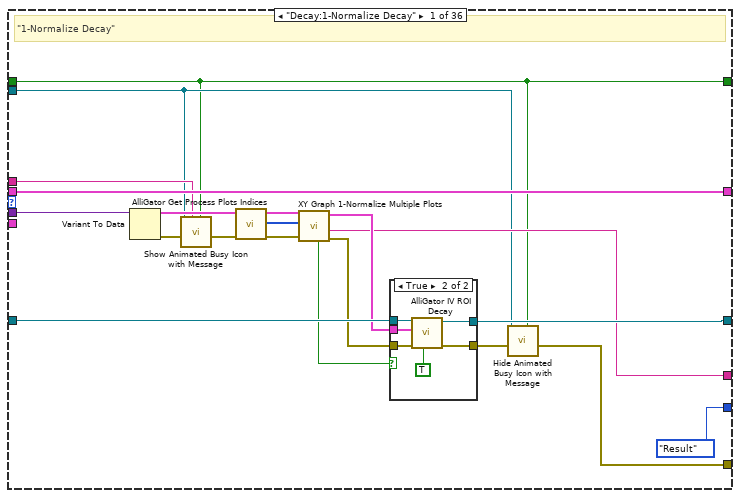
[diagram p2: hidden frame]
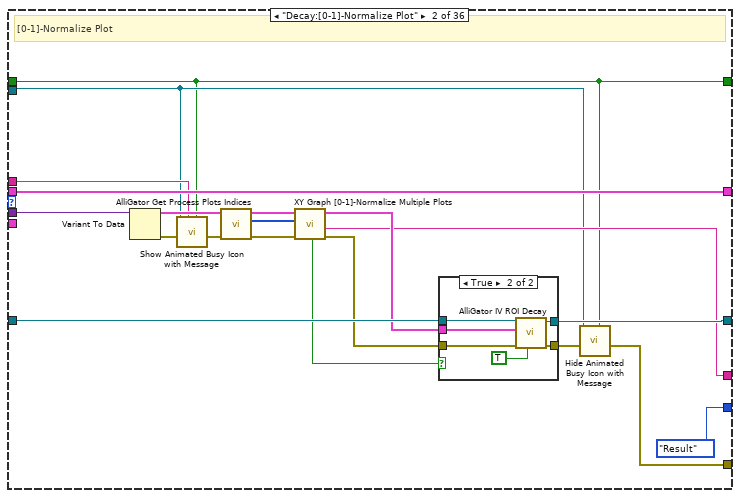
[diagram p4: hidden frame]
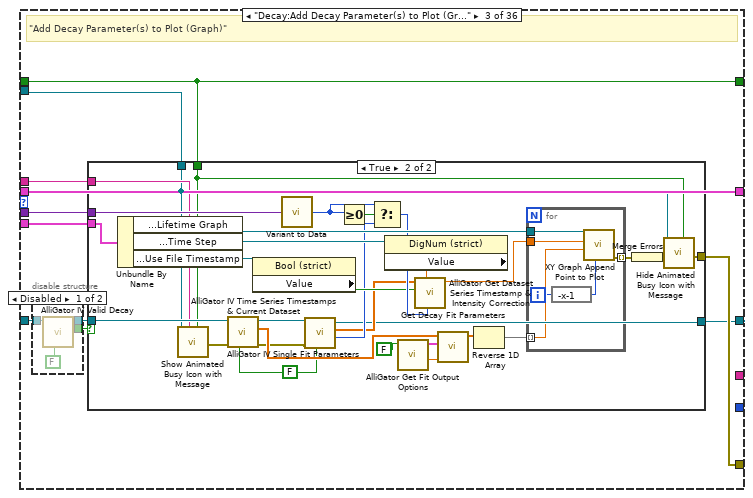
[diagram p6: hidden frame]
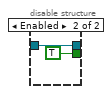
[diagram p7: hidden frame]
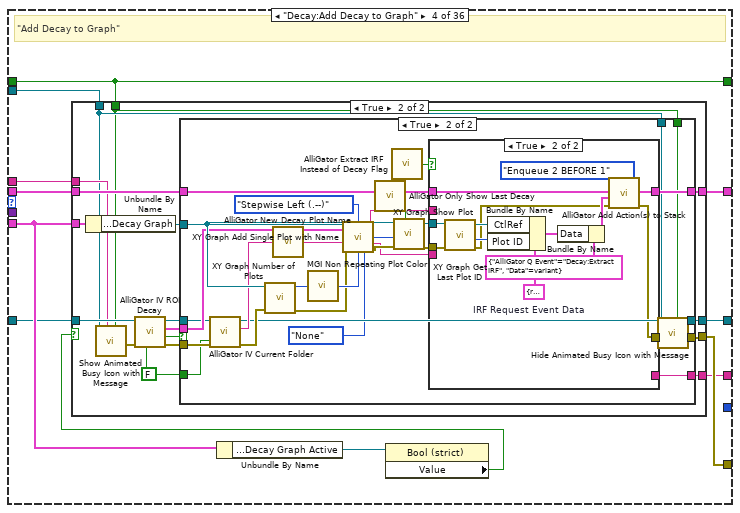
[diagram p9: hidden frame]
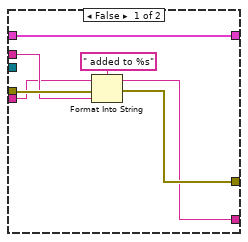
[diagram p12: hidden frame]
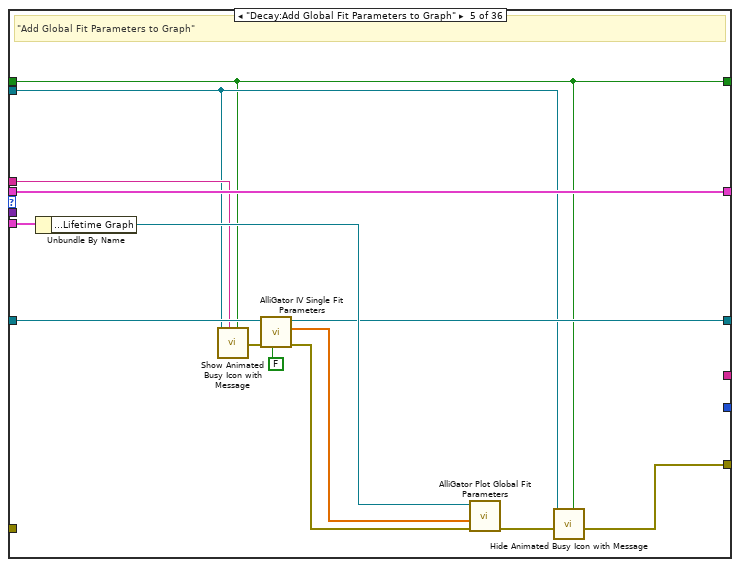
[diagram p13: hidden frame]
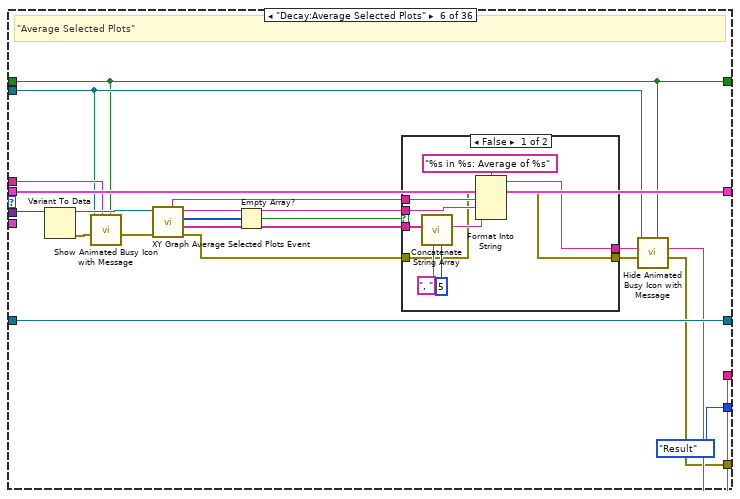
[diagram p14: hidden frame]
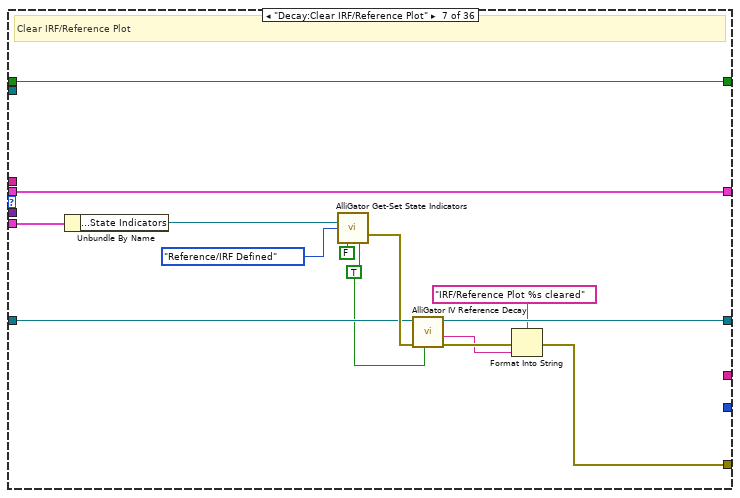
[diagram p16: hidden frame]
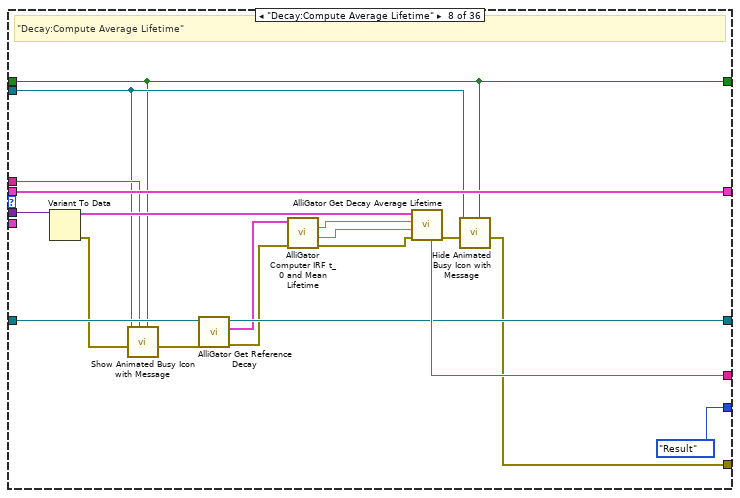
[diagram p17: hidden frame]
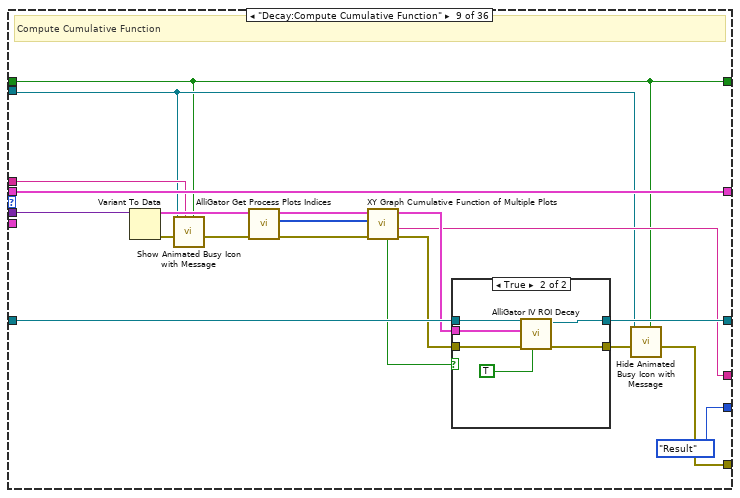
[diagram p18: hidden frame]
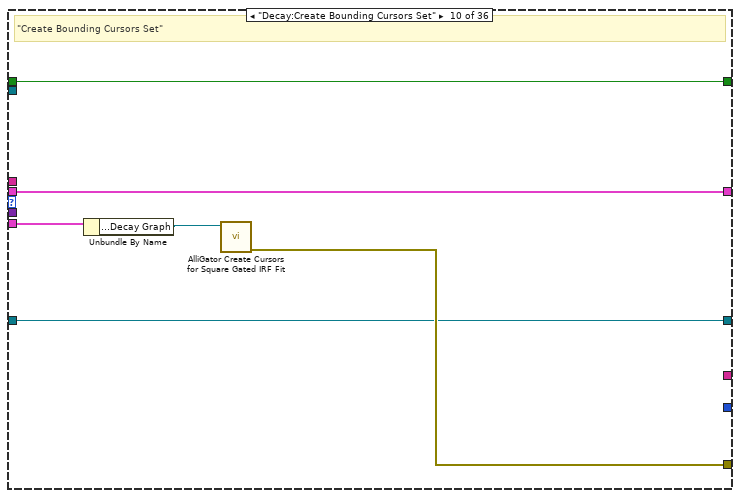
[diagram p20: hidden frame]
diagram:
  # "Author: Xavier Michalet\nCopyright 2025 REGENTS OF THE UNIVERSITY OF CALIFORNIA\n\nRedistribution and use in source and binary forms, with or without modification, are permitted provided that the following conditions are met:\n\n1. Redistributions of source code must retain the above copyright notice, this list of conditions and the following disclaimer.\n\n2. Redistributions in binary form must reproduce the above copyright notice, this list of conditions and the following disclaimer in the documentation and/or other materials provided with the distribution.\n\n3. Neither the name of the copyright holder nor the names of its contributors may be used to endorse or promote products derived from this software without specific prior written permission.\n\nTHIS SOFTWARE IS PROVIDED BY THE COPYRIGHT HOLDERS AND CONTRIBUTORS “AS IS” AND ANY EXPRESS OR IMPLIED WARRANTIES, INCLUDING, BUT NOT LIMITED TO, THE IMPLIED WARRANTIES OF MERCHANTABILITY AND FITNESS FOR A PARTICULAR PURPOSE ARE DISCLAIMED. IN NO EVENT SHALL THE COPYRIGHT HOLDER OR CONTRIBUTORS BE LIABLE FOR ANY DIRECT, INDIRECT, INCIDENTAL, SPECIAL, EXEMPLARY, OR CONSEQUENTIAL DAMAGES (INCLUDING, BUT NOT LIMITED TO, PROCUREMENT OF SUBSTITUTE GOODS OR SERVICES; LOSS OF USE, DATA, OR PROFITS; OR BUSINESS INTERRUPTION) HOWEVER CAUSED AND ON ANY THEORY OF LIABILITY, WHETHER IN CONTRACT, STRICT LIABILITY, OR TORT (INCLUDING NEGLIGENCE OR OTHERWISE) ARISING IN ANY WAY OUT OF THE USE OF THIS SOFTWARE, EVEN IF ADVISED OF THE POSSIBILITY OF SUCH DAMAGE."
  n1 = call "AlliGator Event to String.vi"("AlliGator Q Event"="AlliGator Q Event in") -> ("String"=w9:string)  [unwired: 8 in]
  n2 = case shown="\"Decay:Show Reference Decay/IRF\"" "AlliGator Q Event in" {
    selector: "AlliGator Q Event in" -> [_ _ _ _ _ _ _ _ _ _ _ _ _ _ _ _ _ _ _ _ _ _ _ _ w712 _ _ _ _ _ _ _ _ _ w961 _]
    tunnel: "Data" -> [w37 w65 w83 _ _ w245 _ w287 w308 _ _ w353 _ w375 w423 w443 w463 w510 w542 w559 w576 w599 _ w686 w714 _ w753 w792 _ w844 w877 w891 w913 w938 w963 _]
    tunnel: "AlliGator Q Elements in" -> [w38 w66 w85 w141 w226 w244 w270 w289 w309 w323 w329 w354 w373 w384 w424 w444 w464 w515 w543 w560 w577 w600 w617 w687 w715 w731 w754 w793 w812 w845 w878 w894 w914 w939 w964 w968]
    tunnel: [w38 w66 w85 w140 w226 w244 w270 w289 w309 w323 w329 w354 w373 w383 w424 w444 w464 w515 w543 w560 w577 w600 w616 w687 w715 w730 w754 w793 w812 w845 w878 w894 w914 w939 w964 w968] -> w11
    tunnel: "VI in" -> [w21 w49 w77 w132 w214 w229 _ w273 w292 _ _ w332 _ _ w411 w428 w459 w507 w523 w547 w564 w581 w613 w674 w691 _ w737 w766 _ w823 w857 _ w897 w926 w941 _]
    tunnel: [w20 w48 w76 w131 w213 w228 w269 w272 w291 w322 w328 w331 w365 w385 w410 w427 w461 w506 w522 w546 w563 w580 w615 w673 w690 w734 w736 w765 w811 w822 w856 w893 w896 w925 w940 w967] -> w8
    tunnel: "Script in" -> [w20 w48 w76 w131 w213 w228 w269 w272 w291 w322 w328 w331 w365 w385 w410 w427 w461 w506 w522 w546 w563 w580 w615 w673 w690 w734 w736 w765 w811 w822 w856 w893 w896 w925 w940 w967]
    tunnel: w9 -> [w23 w50 w75 w130 w216 w234 _ w274 w293 _ _ _ _ _ w419 w426 w460 w505 w532 w556 w573 w579 w612 w682 w689 _ w738 w764 _ w824 w855 _ w898 w924 w942 _]
    tunnel: "error in (no error)" -> [_ _ _ _ _ _ _ _ _ _ _ _ _ _ _ _ _ _ _ _ _ _ _ _ _ _ _ _ _ _ _ _ _ _ _ w966]
    tunnel: [w22 w51 w84 w139 w215 w230 w259 w275 w294 w321 w327 w333 w368 w382 w412 w429 w462 w508 w524 w548 w565 w582 w618 w675 w692 w727 w739 w767 w810 w825 w858 w892 w899 w927 w943 w966] -> w1
    tunnel: "AlliGator Ctrl Refnums" -> [_ _ w82 w137 w223 _ w268 _ _ w319 w325 _ w367 w380 _ _ _ _ _ _ _ _ w614 _ _ w732 _ _ w805 _ _ _ _ _ w958 _]
    tunnel: "AlliGator IV DVR in" -> [w34 w62 w79 w135 w222 w233 w263 w282 w306 w318 w324 w341 w366 w378 w418 w441 w455 w514 w530 w554 w572 w595 w611 w681 w709 w725 w750 w788 w804 w839 w872 w889 w911 w936 w956 w965]
    tunnel: [w35 w63 w81 w134 w218 w233 w262 w281 w305 w318 w324 w342 w366 w377 w417 w440 w458 w513 w531 w555 w571 w591 w610 w680 w707 w725 w751 w790 w802 w838 w871 w889 w910 w935 w957 w965] -> w18
    tunnel: [w27 w55 _ w133 _ w232 _ w283 w301 _ _ w340 w364 w376 w413 w436 w457 w511 w526 w550 w567 w590 w609 w676 w710 _ w746 w784 _ w834 w867 w888 w906 w930 w951 _] -> w6
    tunnel: [Text_Format_List."Result" ("Text Format") Text_Format_List."Result" ("Text Format") _ _ _ Text_Format_List."Result" ("Text Format") _ Text_Format_List."Result" ("Text Format") Text_Format_List."Result" ("Text Format") _ _ Text_Format_List."Result" ("Text Format") Text_Format_List."Result" ("Text Format") Text_Format_List."Result" ("Text Format") Text_Format_List."Result" ("Text Format") Text_Format_List."Result" ("Text Format") Text_Format_List."Result" ("Text Format") Text_Format_List."Result" ("Text Format") Text_Format_List."Result" ("Text Format") Text_Format_List."Result" ("Text Format") Text_Format_List."Result" ("Text Format") Text_Format_List."Result" ("Text Format") _ Text_Format_List."Result" ("Text Format") Text_Format_List."Result" ("Text Format") _ Text_Format_List."Result" ("Text Format") Text_Format_List."Result" ("Text Format") _ Text_Format_List."Result" ("Text Format") Text_Format_List."Result" ("Text Format") _ Text_Format_List."Result" ("Text Format") Text_Format_List."Result" ("Text Format") _ _] -> w3
    frame "Decay:1-Normalize Decay" {
      # "\"1-Normalize Decay\""
      n3 = Variant To Data(Variant=w37) -> (data=w31:T28, error out=w36:errorcluster)  [unwired: 2 in]
      n4 = call "Show Animated Busy Icon with Message.vi"("Already active? (F)"=w20, "Message"=w23, "Error In"=w36, "Target VI Refnum"=w21) -> ("Error Out"=w24:errorcluster)  [unwired: 7 in]
      n5 = call "AlliGator Get Process Plots Indices.vi"("error in (no error)"=w24, "Selected Plot Info"=w31) -> ("error out"=w29:errorcluster, "Selected Plots"=w25:i32[], "Selected Plot Info (dup)"=w30:T28)  [unwired: 7 in]
      n6 = call "XY Graph 1-Normalize Multiple Plots.vi"("error in (no error)"=w29, "Selected Plots"=w25, "Selected Plot Info"=w30) -> ("error out"=w33:errorcluster, "1-Normalize Plot Message"=w27:string, "Last 1-Normalized Plot"=w28:cluster{"t Array":dbl[], "IRF Array":dbl[]}, "Single Plot?"=w26:bool)  [unwired: 5 in]
      n7 = case shown="True" w26 {
        tunnel: [w40 w46] -> w35
        tunnel: w34 -> [w40 w45]
        tunnel: w33 -> [w39 w44]
        tunnel: [w39 w43] -> w32
        tunnel: w28 -> [_ w41]
        frame False {
        }
        frame True {
          n8 = call "AlliGator IV ROI Decay.vi"("Get (F)/ Set (T)"=TRUE, "error in (no error)"=w44, "Decay in"=w41, "AlliGator IV DVR in"=w45) -> ("error out"=w43:errorcluster, "AlliGator IV DVR out"=w46:refnum<data-value>)  [unwired: 4 in, 2 out]
        }
      }
      n9 = call "Hide Animated Busy Icon with Message.vi"("Already active? (F)"=w20, "Error In"=w32, "Target VI reference"=w21) -> ("Error Out"=w22:errorcluster)  [unwired: 8 in]
    }
    frame "Decay:[0-1]-Normalize Plot" {
      # "[0-1]-Normalize Plot"
      n10 = Variant To Data(Variant=w65) -> (data=w58:T28, error out=w64:errorcluster)  [unwired: 2 in]
      n11 = call "Show Animated Busy Icon with Message.vi"("Already active? (F)"=w48, "Message"=w50, "Error In"=w64, "Target VI Refnum"=w49) -> ("Error Out"=w52:errorcluster)  [unwired: 7 in]
      n12 = call "AlliGator Get Process Plots Indices.vi"("error in (no error)"=w52, "Selected Plot Info"=w58) -> ("error out"=w59:errorcluster, "Selected Plots"=w53:i32[], "Selected Plot Info (dup)"=w57:T28)  [unwired: 7 in]
      n13 = call "XY Graph [0-1]-Normalize Multiple Plots.vi"("error in (no error)"=w59, "Selected Plots"=w53, "Selected Plot Info"=w57) -> ("error out"=w61:errorcluster, "[0-1]-Normalize Plot Message"=w55:string, "Last [0-1]-Normalized Plot"=w56:cluster{"t Array":dbl[], "IRF Array":dbl[]}, "Single Plot?"=w54:bool)  [unwired: 5 in]
      n14 = case shown="True" w54 {
        tunnel: [w68 w74] -> w63
        tunnel: w62 -> [w68 w73]
        tunnel: w61 -> [w67 w72]
        tunnel: [w67 w71] -> w60
        tunnel: w56 -> [_ w70]
        frame False {
        }
        frame True {
          n15 = call "AlliGator IV ROI Decay.vi"("Get (F)/ Set (T)"=TRUE, "error in (no error)"=w72, "Decay in"=w70, "AlliGator IV DVR in"=w73) -> ("error out"=w71:errorcluster, "AlliGator IV DVR out"=w74:refnum<data-value>)  [unwired: 4 in, 2 out]
        }
      }
      n16 = call "Hide Animated Busy Icon with Message.vi"("Already active? (F)"=w48, "Error In"=w60, "Target VI reference"=w49) -> ("Error Out"=w51:errorcluster)  [unwired: 8 in]
    }
    frame "Decay:Add Decay Parameter(s) to Plot (Graph)" {
      # "\"Add Decay Parameter(s) to Plot (Graph)\""
      n17 = disable-structure shown="Disabled" {
        disable-tunnel: [w88 w91] -> w80
        disable-tunnel: w79 -> [w87 w91]
        disable-tunnel: [w86 TRUE ("Valid Decay")] -> w78
        frame Disabled {
          n18 = call "AlliGator IV Valid Decay.vi"("Get (F)/ Set (T)"=FALSE, "AlliGator IV DVR in"=w87) -> ("Valid Decay"=w86:bool, "AlliGator IV DVR out"=w88:refnum<data-value>)  [unwired: 7 in, 1 out]
        }
        frame Enabled {
        }
      }
      n19 = case shown="True" w78 {
        tunnel: [_ w95] -> w84
        tunnel: w83 -> [_ w117]
        tunnel: w82 -> [_ w110]
        tunnel: [w92 w100] -> w81
        tunnel: w80 -> [w92 w98]
        tunnel: w77 -> [_ w94]
        tunnel: w76 -> [_ w93]
        tunnel: w75 -> [_ w96]
        frame False {
        }
        frame True {
          w99 = FALSE ("Get (F)/ Set (T)")
          n20 = Unbundle By Name(w110) -> ("Registered Events Ctrl Refnums.Lifetime Graph"=w118:refnum<vi>, "Other AlliGator Ctrl Refnums.Time Step"=w109:refnum<vi>, "Other AlliGator Ctrl Refnums.Use File Timestamp"=w107:refnum<vi>)
          n21 = call "Show Animated Busy Icon with Message.vi"("Already active? (F)"=w93, "Message"=w96, "Target VI Refnum"=w94) -> ("Error Out"=w97:errorcluster)  [unwired: 8 in]
          n22 = call "AlliGator IV Single Fit Parameters.vi"("Get (F)/ Set (T)"=w99, "error in (no error)"=w97, "AlliGator IV DVR in"=w98) -> ("error out"=w102:errorcluster, "[Single Decay Fit Parameter]"=w105:dbl[], "AlliGator IV DVR out"=w104:refnum<data-value>)  [unwired: 6 in]
          n23 = property class="Bool (strict)"(reference=w107) -> ("Value"=w106:bool)  [unwired: 1 in, 2 out]
          n24 = call-poly "Variant to Data.vi"("Variant"=w117) -> ("Value"=w115:i32)  [unwired: 8 in]
          n25 = call "AlliGator IV Time Series Timestamps & Current Dataset.vi"("Get (F)/ Set"=w99, "error in (no error)"=w102, "AlliGator IV DVR in"=w104) -> ("Current Dataset"=w103:i32, "[Time-Series Timestamps]"=w101:dbl[], "AlliGator IV DVR out"=w100:refnum<data-value>)  [unwired: 5 in, 1 out]
          n26 = Greater Or Equal To 0?(x=w115) -> (x >= 0?=w116:bool)
          n27 = Select(t=w115, s=w116, f=w103) -> (s? t:f=w114:i32)
          n28 = property class="DigNum (strict)"(reference=w109) -> ("Value"=w108:dbl[unit])  [unwired: 1 in, 2 out]
          n29 = call "AlliGator Get Fit Output Options.vi"("All Parameters?"=FALSE) -> ("Laser Period"=w111:dbl, "Decay Fit Output Options"=w113:T29)  [unwired: 8 in, 1 out]
          n30 = call "AlliGator Get Dataset Series Timestamp & Intensity Correction.vi"("Current Data Set"=w114, "Time Step"=w108, "Use File Timestamp"=w106, "Dataset Series Timestamps"=w101) -> ("Time Stamp (s)"=w123:dbl)  [unwired: 6 in, 1 out]
          n31 = call "Get Decay Fit Parameters.vi"("Laser Period"=w111, "Decay Fit Output Options"=w113, "Decay Fit Parameters"=w105) -> ("Displayed Decay Fits Parameters"=w122:dbl[])  [unwired: 7 in, 1 out]
          n32 = Reverse 1D Array(array=w122) -> (reversed array=w121:dbl[])
          n33 = for {
            tunnel: w118 -> [w129]
            tunnel: w123 -> [w128]
            tunnel: w121 -> [w127] mode=indexing
            tunnel: [w124] -> w120 mode=indexing
            i -> [w126]
            n34 = expression code="-x-1"(w126) -> (w125:i32)
            n35 = call "XY Graph Append Point to Plot.vi"("Plot ID (-1: last)"=w125, "y"=w127, "x"=w128, "XYGraph in"=w129) -> ("error out"=w124:errorcluster)  [unwired: 4 in, 3 out]
          }
          n36 = Merge Errors(w120) -> (w119:errorcluster)
          n37 = call "Hide Animated Busy Icon with Message.vi"("Already active? (F)"=w93, "Error In"=w119, "Target VI reference"=w94) -> ("Error Out"=w95:errorcluster)  [unwired: 8 in]
        }
      }
    }
    frame "Decay:Add Decay to Graph" {
      # "\"Add Decay to Graph\""
      n38 = Unbundle By Name(w137) -> ("Other AlliGator Ctrl Refnums.Decay Graph Active"=w138:refnum<vi>)
      n39 = property class="Bool (strict)"(reference=w138) -> ("Value"=w136:bool)  [unwired: 1 in, 2 out]
      n40 = case shown="True" w136 {
        tunnel: w141 -> [w143 w160]
        tunnel: [w143 w159] -> w140
        tunnel: w137 -> [_ w158]
        tunnel: [_ w156] -> w139
        tunnel: w135 -> [w142 w155]
        tunnel: [w142 w150] -> w134
        tunnel: [_ w149] -> w133
        tunnel: w132 -> [_ w145]
        tunnel: w131 -> [_ w144]
        tunnel: w130 -> [_ w146]
        frame False {
        }
        frame True {
          w151 = FALSE ("Get (F)/ Set (T)")
          n41 = Unbundle By Name(w158) -> ("Registered Events Ctrl Refnums.Decay Graph"=w157:refnum<vi>)
          n42 = call "Show Animated Busy Icon with Message.vi"("Already active? (F)"=w144, "Message"=w146, "Target VI Refnum"=w145) -> ("Error Out"=w147:errorcluster)  [unwired: 8 in]
          n43 = call "AlliGator IV ROI Decay.vi"("Get (F)/ Set (T)"=w151, "error in (no error)"=w147, "AlliGator IV DVR in"=w155) -> ("error out"=w152:errorcluster, "Valid Decay?"=w148:bool, "Decay out"=w154:cluster{"t Array":dbl[], "IRF Array":dbl[]}, "AlliGator IV DVR out"=w153:refnum<data-value>)  [unwired: 5 in]
          n44 = case shown="True" w148 {
            tunnel: w160 -> [w163 w192]
            tunnel: [w163 w191] -> w159
            tunnel: w157 -> [_ w181]
            tunnel: [w161 w168] -> w156
            tunnel: w154 -> [_ w178]
            tunnel: w153 -> [w162 w177]
            tunnel: w152 -> [w161 w176]
            tunnel: w151 -> [_ w174]
            tunnel: [w162 w172] -> w150
            tunnel: [_ w169] -> w149
            tunnel: w145 -> [_ w167]
            tunnel: w144 -> [_ w166]
            frame False {
            }
            frame True {
              n45 = call "AlliGator IV Current Folder.vi"("Get (F)/ Set (T)"=w174, "error in (no error)"=w176, "AlliGator IV DVR in"=w177) -> ("error out"=w173:errorcluster, "Current Folder"=w175:string, "AlliGator IV DVR out"=w172:refnum<data-value>)  [unwired: 6 in]
              n46 = call "XY Graph Number of Plots.vi"("Error In"=w173, "XYGraph in"=w181) -> ("Error Out"=w180:errorcluster, "# Plots"=w182:i32)  [unwired: 8 in]
              n47 = call "AlliGator New Decay Plot Name.vi"("Current Folder"=w175) -> ("New Decay Name"=w189:string)  [unwired: 8 in]
              n48 = call <userlib>:"MGI Non Repeating Plot Color.vi"("Plot #"=w182) -> ("Color"=w183:u32)
              n49 = call "XY Graph Add Single Plot with Name.vi"("XYGraph Ref in"=w181, "Plot Interpolation (Previous Plot's Style)"=LabVIEW_Plot_Interpolation."Stepwise Left (.--)", "Plot"=w178, "Plot Name (\"Plot\")"=w189, "error in (no error)"=w180, "Plot Color (Default)"=w183, "Point Style (Dot)"=Plot_Point_Style."None") -> ("XY Graph Caption (or Label)"=w170:string, "Plot Index"=w187:i32, "Plot Name"=w171:string, "error out"=w188:errorcluster)  [unwired: 5 in]
              n50 = call "AlliGator Only Show Last Decay.vi"() -> ("Show Last Decay Only?"=w186:bool)
              n51 = call "AlliGator Extract IRF Instead of Decay Flag.vi"() -> ("Extract IRF instead of Decay?"=w190:bool)
              n52 = call "XY Graph Show Plot.vi"("Hide All Other Plots (F)"=w186, "error in (no error)"=w188, "Selected Plot Index"=w187, "XY Graph in"=w181) -> ("error out"=w184:errorcluster, "XY Graph out"=w185:T24)  [unwired: 6 in]
              n53 = case shown="True" w190 {
                tunnel: w185 -> [_ w207]
                tunnel: w192 -> [w199 w205]
                tunnel: [w199 w202] -> w191
                tunnel: w184 -> [w198 w206]
                tunnel: [w197 w200] -> w179
                tunnel: w171 -> [w193 _]
                tunnel: w170 -> [w196 _]
                tunnel: [w194 _] -> w169
                frame False {
                  n54 = Format Into String(format string=" added to %s", initial string=w193, error in=w198, w196) -> (resulting string=w194:string, error out=w197:errorcluster)
                }
                frame True {
                  w208 = T32 {"CtlRef"=refnum, "Coords"={"Horizontal"=0, "Vertical"=0}, "Plot ID"=0}  # IRF Request Event Data
                  n55 = call "XY Graph Get Last Plot ID.vi"("error in (no error)"=w206, "XYGraph in"=w207) -> ("error out"=w203:errorcluster, "Last Plot ID"=w209:i32, "XYGraph out"=w210:refnum<vi>)  [unwired: 7 in]
                  n56 = Bundle By Name(cluster=w208, "CtlRef"=w210, "Plot ID"=w209) -> (w211:T32)
                  n57 = Bundle By Name(cluster=T6 {"AlliGator Q Event"=enum."Decay:Extract IRF", "Data"=variant} ("element"), "Data"=w211) -> (w204:T6)
                  n58 = call-poly "AlliGator Add Action(s) to Stack.vi"("Elements Order in Action Stack (Default: 2 BEFORE 1)"=Alligator_Elements_Order_in_Action_Stack."Enqueue 2 BEFORE 1", "Error In"=w203, "Alligator Atomic Action"=w204, "Alligator Queue Element 1"=w205) -> ("Error Out"=w200:errorcluster, "Alligator Queue Element 1 (+ 2)"=w202:T6[])  [unwired: 6 in]
                }
              }
              n59 = call "Hide Animated Busy Icon with Message.vi"("Already active? (F)"=w166, "Error In"=w179, "Target VI reference"=w167) -> ("Error Out"=w168:errorcluster)  [unwired: 8 in]
            }
          }
        }
      }
    }
    frame "Decay:Add Global Fit Parameters to Graph" {
      # "\"Add Global Fit Parameters to Graph\""
      n60 = Unbundle By Name(w223) -> ("Registered Events Ctrl Refnums.Lifetime Graph"=w224:refnum<vi>)
      n61 = call "Show Animated Busy Icon with Message.vi"("Already active? (F)"=w213, "Message"=w216, "Target VI Refnum"=w214) -> ("Error Out"=w217:errorcluster)  [unwired: 8 in]
      n62 = call "AlliGator IV Single Fit Parameters.vi"("Get (F)/ Set (T)"=FALSE, "error in (no error)"=w217, "AlliGator IV DVR in"=w222) -> ("error out"=w220:errorcluster, "[Single Decay Fit Parameter]"=w221:dbl[], "AlliGator IV DVR out"=w218:refnum<data-value>)  [unwired: 6 in]
      n63 = call "AlliGator Plot Global Fit Parameters.vi"("Error In"=w220, "Best Fit Parameters"=w221, "XYGraph in"=w224) -> ("Error Out"=w225:errorcluster)  [unwired: 8 in]
      n64 = call "Hide Animated Busy Icon with Message.vi"("Already active? (F)"=w213, "Error In"=w225, "Target VI reference"=w214) -> ("Error Out"=w215:errorcluster)  [unwired: 8 in]
    }
    frame "Decay:Average Selected Plots" {
      # "\"Average Selected Plots\""
      n65 = Variant To Data(Variant=w245) -> (data=w240:refnum<vi>, error out=w238:errorcluster)  [unwired: 2 in]
      n66 = call "Show Animated Busy Icon with Message.vi"("Already active? (F)"=w228, "Message"=w234, "Error In"=w238, "Target VI Refnum"=w229) -> ("Error Out"=w239:errorcluster)  [unwired: 7 in]
      n67 = call "XY Graph Average Selected Plots Event.vi"("Error In"=w239, "XYGraph Ref"=w240) -> ("Error Out"=w231:errorcluster, "Averaged Plot Names"=w243:string[], "Averaged Plot Indices"=w242:i32[], "Graph Label"=w237:string, "Plot Name"=w236:string)  [unwired: 5 in]
      n68 = Empty Array?(array=w242) -> (empty?=w241:bool)
      n69 = case shown="False" w241 {
        tunnel: w243 -> [w253 _]
        tunnel: w237 -> [w254 _]
        tunnel: w236 -> [w250 _]
        tunnel: w231 -> [w247 w256]
        tunnel: [w249 w256] -> w235
        tunnel: [w246 _] -> w232
        frame False {
          n70 = call "Concatenate String Array.vi"("Max Number of Elements (None: -1)"=5 ("Max Number of Elements (None: 1)"), "Separator (TAB)"=", ", "String Array"=w253) -> ("Formatted String"=w251:string)  [unwired: 8 in]
          n71 = Format Into String(format string="%s in %s: Average of %s", error in=w247, w250, w254, w251) -> (resulting string=w246:string, error out=w249:errorcluster)  [unwired: 1 in]
        }
        frame True {
        }
      }
      n72 = call "Hide Animated Busy Icon with Message.vi"("Already active? (F)"=w228, "Error In"=w235, "Target VI reference"=w229) -> ("Error Out"=w230:errorcluster)  [unwired: 8 in]
    }
    frame "Decay:Clear IRF/Reference Plot" {
      w260 = TRUE ("Set (T)/Get")
      # "Clear IRF/Reference Plot"
      n73 = Unbundle By Name(w268) -> ("Other AlliGator Ctrl Refnums.State Indicators"=w265:refnum<vi>)
      n74 = call "AlliGator Get-Set State Indicators.vi"("State Indicators Refnum"=w265, "AlliGator State Indicators List"=AlliGator_State_Indicators_List."Reference/IRF Defined", "ON/OFF"=FALSE, "Set (T)/Get"=w260) -> ("Error Out"=w264:errorcluster)  [unwired: 9 in, 2 out]
      n75 = call "AlliGator IV Reference Decay.vi"("Get (F)/ Set (T)"=w260, "Error In"=w264, "AlliGator IV DVR in"=w263) -> ("Error Out"=w261:errorcluster, "Reference Decay Plot Name"=w258:string, "AlliGator IV DVR out"=w262:refnum<data-value>)  [unwired: 5 in, 1 out]
      n76 = Format Into String(format string="IRF/Reference Plot %s cleared", error in=w261, w258) -> (error out=w259:errorcluster)  [unwired: 1 in, 1 out]
    }
    frame "Decay:Compute Average Lifetime" {
      # "\"Decay:Compute Average Lifetime\""
      n77 = Variant To Data(Variant=w287) -> (data=w286:T28, error out=w279:errorcluster)  [unwired: 2 in]
      n78 = call "Show Animated Busy Icon with Message.vi"("Already active? (F)"=w272, "Message"=w274, "Error In"=w279, "Target VI Refnum"=w273) -> ("Error Out"=w276:errorcluster)  [unwired: 7 in]
      n79 = call "AlliGator Get Reference Decay.vi"("Error In"=w276, "Data Value Reference in"=w282) -> ("Error Out"=w278:errorcluster, "Reference Decay"=w280:cluster{"t Array":dbl[], "I Array":dbl[]}, "Data Value Reference out"=w281:refnum<data-value>)  [unwired: 7 in]
      n80 = call "AlliGator Computer IRF t_0 and Mean Lifetime.vi"("error in"=w278, "Reference Decay"=w280) -> ("error out"=w285:errorcluster, "t_0"=w284:dbl, "<tau>_IRF"=w277:dbl)  [unwired: 7 in]
      n81 = call "AlliGator Get Decay Average Lifetime.vi"("error in (no error)"=w285, "t_0_IRF"=w284, "<tau>_IRF"=w277, "Selected Plot Info"=w286) -> ("Error Out"=w288:errorcluster, "Message"=w283:string)  [unwired: 6 in]
      n82 = call "Hide Animated Busy Icon with Message.vi"("Already active? (F)"=w272, "Error In"=w288, "Target VI reference"=w273) -> ("Error Out"=w275:errorcluster)  [unwired: 8 in]
    }
    frame "Decay:Compute Cumulative Function" {
      # "Compute Cumulative Function"
      n83 = Variant To Data(Variant=w308) -> (data=w299:T28, error out=w307:errorcluster)  [unwired: 2 in]
      n84 = call "Show Animated Busy Icon with Message.vi"("Already active? (F)"=w291, "Message"=w293, "Error In"=w307, "Target VI Refnum"=w292) -> ("Error Out"=w295:errorcluster)  [unwired: 7 in]
      n85 = call "AlliGator Get Process Plots Indices.vi"("error in (no error)"=w295, "Selected Plot Info"=w299) -> ("error out"=w300:errorcluster, "Selected Plots"=w296:i32[], "Selected Plot Info (dup)"=w298:T28)  [unwired: 7 in]
      n86 = call "XY Graph Cumulative Function of Multiple Plots.vi"("error in (no error)"=w300, "Selected Plots"=w296, "Selected Plot Info"=w298) -> ("error out"=w303:errorcluster, "Cumulative Function Plot Message"=w301:string, "Last Cumulative Function Plot"=w304:cluster{"t Array":dbl[], "IRF Array":dbl[]}, "Single Plot?"=w297:bool)  [unwired: 5 in]
      n87 = case shown="True" w297 {
        tunnel: w306 -> [w311 w317]
        tunnel: [w311 w316] -> w305
        tunnel: w304 -> [_ w315]
        tunnel: w303 -> [w310 w314]
        tunnel: [w310 w313] -> w302
        frame False {
        }
        frame True {
          n88 = call "AlliGator IV ROI Decay.vi"("Get (F)/ Set (T)"=TRUE, "error in (no error)"=w314, "Decay in"=w315, "AlliGator IV DVR in"=w317) -> ("error out"=w313:errorcluster, "AlliGator IV DVR out"=w316:refnum<data-value>)  [unwired: 4 in, 2 out]
        }
      }
      n89 = call "Hide Animated Busy Icon with Message.vi"("Already active? (F)"=w291, "Error In"=w302, "Target VI reference"=w292) -> ("Error Out"=w294:errorcluster)  [unwired: 8 in]
    }
    frame "Decay:Create Bounding Cursors Set" {
      # "\"Create Bounding Cursors Set\""
      n90 = Unbundle By Name(w319) -> ("Registered Events Ctrl Refnums.Decay Graph"=w320:refnum<vi>)
      n91 = call "AlliGator Create Cursors for Square Gated IRF Fit.vi"("Decay Graph"=w320) -> ("Error Out"=w321:errorcluster)  [unwired: 9 in, 1 out]
    }
    frame "Decay:Create Head & Tail Bounding Cursors" {
      # "Create Head & Tail Bounding Cursors"
      n92 = Unbundle By Name(w325) -> ("Registered Events Ctrl Refnums.Decay Graph"=w326:refnum<vi>)
      n93 = call "AlliGator Create Head & Tail Bounding Cursors.vi"("Decay Graph"=w326) -> ("Error Out"=w327:errorcluster)  [unwired: 9 in, 1 out]
    }
    frame "Decay:Denoise Plot" {
      # "\"Denoise Plot\""
      n94 = Variant To Data(Variant=w353) -> (data=w338:T28, error out=w352:errorcluster)  [unwired: 2 in]
      n95 = call "Show Animated Busy Icon with Message.vi"("Already active? (F)"=w331, "Error In"=w352, "Target VI Refnum"=w332) -> ("Error Out"=w334:errorcluster)  [unwired: 8 in]
      n96 = call "AlliGator Settings Storage.vi"("AlliGator Settings List"=AlliGator_Settings_List."Fluorescence Decay_Advanced Analysis:Wavelet Analysis Options") -> ("Error Out"=w348:errorcluster, "Variant Data out"=w350:variant)  [unwired: 9 in]
      n97 = call "AlliGator Get Process Plots Indices.vi"("error in (no error)"=w334, "Selected Plot Info"=w338) -> ("error out"=w339:errorcluster, "Selected Plots"=w336:i32[], "Selected Plot Info (dup)"=w337:T28)  [unwired: 7 in]
      n98 = Variant To Data(error in=w348, Variant=w350) -> (data=w349:T33, error out=w346:errorcluster)  [unwired: 1 in]
      n99 = Merge Errors(w346, w339) -> (w347:errorcluster)
      n100 = call "XY Graph Denoise Multiple Plots.vi"("Wavelet Analysis Options"=w349, "error in (no error)"=w347, "Selected Plots"=w336, "Selected Plot Info"=w337) -> ("error out"=w344:errorcluster, "Denoised Plot Message"=w340:string, "Last Denoised Plot"=w345:cluster{"t Array":dbl[], "IRF Array":dbl[]}, "Single Plot?"=w335:bool)  [unwired: 4 in]
      n101 = case shown="False" w335 {
        tunnel: w345 -> [_ w362]
        tunnel: w344 -> [w355 w361]
        tunnel: [w355 w360] -> w343
        tunnel: [w356 w359] -> w342
        tunnel: w341 -> [w356 w358]
        frame False {
        }
        frame True {
          n102 = call "AlliGator IV ROI Decay.vi"("Get (F)/ Set (T)"=TRUE, "error in (no error)"=w361, "Decay in"=w362, "AlliGator IV DVR in"=w358) -> ("error out"=w360:errorcluster, "AlliGator IV DVR out"=w359:refnum<data-value>)  [unwired: 4 in, 2 out]
        }
      }
      n103 = call "Hide Animated Busy Icon with Message.vi"("Already active? (F)"=w331, "Error In"=w343, "Target VI reference"=w332) -> ("Error Out"=w333:errorcluster)  [unwired: 8 in]
    }
    frame "Decay:Export Bounding Cursors Definition to Notebook" {
      # "Export Bounding Cursors Definition to Notebook"
      n104 = Unbundle By Name(w367) -> ("Registered Events Ctrl Refnums.Decay Graph"=w369:refnum<vi>)
      n105 = call "AlliGator Get Square Gated IRF Analysis Cursors.vi"("XYGraph in"=w369) -> ("Error Out"=w372:errorcluster, "Cursor Names Array"=w370:string[], "Cursor Positions Array"=w371:dbl[])  [unwired: 7 in, 1 out]
      n106 = call "AlliGator Square Gated IRF Fit Cursors String.vi"("Error In"=w372, "Cursor Positions Array"=w371, "Cursor Names Array"=w370) -> ("Error Out"=w368:errorcluster, "Message"=w364:string)  [unwired: 7 in]
    }
    frame "Decay:Export Decay to Phasor Graph" {
      # "\"Export Decay to Phasor Graph\""
      n107 = Unbundle By Name(w380) -> ("Phasor Graph Ctrl Refnums.Phasor Graph Active"=w381:refnum<vi>)
      n108 = property class="Bool (strict)"(reference=w381) -> ("Value"=w379:bool)  [unwired: 1 in, 2 out]
      n109 = case shown="True" w379 {
        tunnel: w384 -> [w388 w405]
        tunnel: [w388 w404] -> w383
        tunnel: [_ w401] -> w382
        tunnel: w378 -> [w386 w396]
        tunnel: [w386 w394] -> w377
        tunnel: [_ w393] -> w376
        tunnel: w375 -> [_ w391]
        frame False {
          n110 = One Button Dialog(message="Phasor Graph inactive!") -> ()  [unwired: 1 in, 1 out]
          n111 = call "Play Error Sound.vi"() -> ()  [unwired: 27 in, 1 out]
        }
        frame True {
          w398 = T34 {"Global Rectangle"=[], "Contours"=[{"ID"=enum."External", "Type"=1, "Coordinates"=[]}]}  # Dummy Point
          n112 = Variant To Data(Variant=w391) -> (data=w389:T28, error out=w390:errorcluster)  [unwired: 2 in]
          n113 = call "XY Graph Get Selected Plot.vi"("error in (no error)"=w390, "Selected Plot Info"=w389) -> ("error out"=w395:errorcluster, "Plot Name"=w400:string, "Plot"=w407:T35)  [unwired: 4 in, 3 out]
          n114 = call "AlliGator Get ROI Decay.vi"("error in (no error)"=w395, "Decay"=w407, "ROI Descriptor"=w398, "AlliGator Internal Variables DVR"=w396) -> ("Error Out"=w402:errorcluster, "AlliGator Internal Variables DVR"=w394:refnum<data-value>, "Message"=w392:string)  [unwired: 2 in, 3 out]
          n115 = Format Into String(format string="\n%s's phasor added to Phasor Graph", initial string=w392, error in=w402, w400) -> (resulting string=w393:string, error out=w397:errorcluster)
          n116 = call-poly "AlliGator Add Action(s) to Stack.vi"("Elements Order in Action Stack (Default: 2 BEFORE 1)"=Alligator_Elements_Order_in_Action_Stack."Enqueue 2 BEFORE 1", "Error In"=w397, "Alligator Queue Element 2"=T6[] [{"AlliGator Q Event"=enum."Phasor Graph:Create New Phasor Plot Dialog", "Data"=variant}, {"AlliGator Q Event"=enum."Phasor Graph:Get Phasor Value", "Data"=variant}] ("Alligator Atomic Action"), "Alligator Queue Element 1"=w405) -> ("Error Out"=w401:errorcluster, "Alligator Queue Element 1 (+ 2)"=w404:T6[])  [unwired: 6 in]
        }
      }
    }
    frame "Decay:Extract IRF" {
      # "\"Extract IRF\""
      n117 = Variant To Data(Variant=w423) -> (data=w421:T28, error out=w422:errorcluster)  [unwired: 2 in]
      n118 = call "Show Animated Busy Icon with Message.vi"("Already active? (F)"=w410, "Message"=w419, "Error In"=w422, "Target VI Refnum"=w411) -> ("Error Out"=w420:errorcluster)  [unwired: 7 in]
      n119 = call "AlliGator Get IRF from Decay v2.vi"("error in (no error)"=w420, "Selected Plot Info"=w421) -> ("Error Out"=w409:errorcluster, "Message"=w413:string, "Extracted IRF"=w415:cluster{"t Array":dbl[], "IRF Array":dbl[]})  [unwired: 7 in]
      n120 = call "AlliGator IV ROI Decay.vi"("Get (F)/ Set (T)"=TRUE, "error in (no error)"=w409, "Decay in"=w415, "AlliGator IV DVR in"=w418) -> ("error out"=w416:errorcluster, "AlliGator IV DVR out"=w417:refnum<data-value>)  [unwired: 4 in, 2 out]
      n121 = call "Hide Animated Busy Icon with Message.vi"("Already active? (F)"=w410, "Error In"=w416, "Target VI reference"=w411) -> ("Error Out"=w412:errorcluster)  [unwired: 8 in]
    }
    frame "Decay:Extrapolate Decay" {
      # "\"Extrapolate Decay\""
      n122 = Variant To Data(Variant=w443) -> (data=w434:T28, error out=w442:errorcluster)  [unwired: 2 in]
      n123 = call "Show Animated Busy Icon with Message.vi"("Already active? (F)"=w427, "Message"=w426, "Error In"=w442, "Target VI Refnum"=w428) -> ("Error Out"=w430:errorcluster)  [unwired: 7 in]
      n124 = call "AlliGator Get Process Plots Indices.vi"("error in (no error)"=w430, "Selected Plot Info"=w434) -> ("error out"=w435:errorcluster, "Selected Plots"=w432:i32[], "Selected Plot Info (dup)"=w433:T28)  [unwired: 7 in]
      n125 = call "AlliGator Extrapolate Multiple Plots.vi"("error in (no error)"=w435, "Selected Plots"=w432, "Selected Plot Info"=w433) -> ("error out"=w438:errorcluster, "Extrapolated Decay Message"=w436:string, "Last Extrapolated Decay"=w439:cluster{"t Array":dbl[], "IRF Array":dbl[]}, "Single Plot?"=w431:bool)  [unwired: 5 in]
      n126 = case shown="True" w431 {
        tunnel: w441 -> [w446 w452]
        tunnel: [w446 w451] -> w440
        tunnel: w439 -> [_ w450]
        tunnel: w438 -> [w445 w449]
        tunnel: [w445 w448] -> w437
        frame False {
        }
        frame True {
          n127 = call "AlliGator IV ROI Decay.vi"("Get (F)/ Set (T)"=TRUE, "error in (no error)"=w449, "Decay in"=w450, "AlliGator IV DVR in"=w452) -> ("error out"=w448:errorcluster, "AlliGator IV DVR out"=w451:refnum<data-value>)  [unwired: 4 in, 2 out]
        }
      }
      n128 = call "Hide Animated Busy Icon with Message.vi"("Already active? (F)"=w427, "Error In"=w437, "Target VI reference"=w428) -> ("Error Out"=w429:errorcluster)  [unwired: 8 in]
    }
    frame "Decay:Fit Decay" {
      # "\"Fit Decay\""
      n129 = disable-structure shown="Enabled" {
        disable-tunnel: [w468 w470] -> w456
        disable-tunnel: w455 -> [w467 w470]
        disable-tunnel: [w465 TRUE ("Valid Decay")] -> w454
        frame Disabled {
          n130 = call "AlliGator IV Valid Decay.vi"("Get (F)/ Set (T)"=FALSE, "AlliGator IV DVR in"=w467) -> ("Valid Decay"=w465:bool, "AlliGator IV DVR out"=w468:refnum<data-value>)  [unwired: 7 in, 1 out]
        }
        frame Enabled {
        }
      }
      n131 = case shown="True" w454 {
        tunnel: w463 -> [_ w502]
        tunnel: [_ w501] -> w462
        tunnel: w461 -> [_ w500]
        tunnel: w460 -> [_ w499]
        tunnel: w459 -> [_ w498]
        tunnel: [w471 w493] -> w458
        tunnel: [_ w492] -> w457
        tunnel: w456 -> [w471 w491]
        frame False {
        }
        frame True {
          w486 = "Abort Fit" ("Abort Button Name (Abort)")
          n132 = call "AlliGator Check Decay Reference.vi"("AlliGator Internal Variables DVR"=w491) -> ("Error Out"=w496:errorcluster, "Reference Decay"=w474:cluster{"t Array":dbl[], "I Array":dbl[]}, "AlliGator Internal Variables DVR"=w497:refnum<data-value>)  [unwired: 3 in, 5 out]
          n133 = call "AlliGator IV ROI Decay.vi"("Get (F)/ Set (T)"=FALSE, "error in (no error)"=w496, "AlliGator IV DVR in"=w497) -> ("error out"=w495:errorcluster, "Decay out"=w472:cluster{"t Array":dbl[], "IRF Array":dbl[]}, "AlliGator IV DVR out"=w494:refnum<data-value>)  [unwired: 5 in, 1 out]
          n134 = Variant To Data(error in=w495, type=T23 {"Multiplot XY Graph"=refnum, "Mouse Coordinates"={"Horizontal"=0, "Vertical"=0}, "Plot Index"=-1, "Flag"=FALSE} ("Selected Plot Info + Flag"), Variant=w502) -> (data=w485:T23, error out=w490:errorcluster)
          n135 = call "Show Animated Busy Icon with Message and Abort Button.vi"("Already active? (F)"=w500, "Message"=w499, "Target VI reference"=w498, "Error In"=w490, "Abort Button Name (Abort)"=w486) -> ("Error Out"=w479:errorcluster)  [unwired: 14 in]
          n136 = call "AlliGator Get Fit Options & Parameters.vi"("error in (no error)"=w479, "Reset Fit Options & Parameters"=TRUE) -> ("error out"=w478:errorcluster, "Use Legacy Fitting Approach"=w477:bool, "Decay Fit Options & Parameters"=w476:T36)  [unwired: 7 in]
          n137 = call "AlliGator Fit Decay.vi"("Selected Plot Info + Flag"=w485, "Decay Fit Options & Parameters"=w476, "Current Decay"=w472, "Reference Decay"=w474, "error in (no error)"=w478, "Use Legacy Fitting Approach"=w477) -> ("Best Fit Parameters (All)"=w489:dbl[], "R^2"=w488:dbl, "Reduced Chi^2"=w487:dbl, "Fit Output Message"=w492:string, "Error Out"=w481:errorcluster)  [unwired: 1 in, 4 out]
          n138 = Build Array (concatenate)(w489, w488, w487) -> (w483:dbl[])
          n139 = call "AlliGator IV Single Fit Parameters.vi"("Get (F)/ Set (T)"=TRUE, "error in (no error)"=w481, "[Single Decay Fit Parameter]"=w483, "AlliGator IV DVR in"=w494) -> ("error out"=w480:errorcluster, "AlliGator IV DVR out"=w493:refnum<data-value>)  [unwired: 5 in, 1 out]
          n140 = call "Hide Animated Busy Icon with Message and Abort Button.vi"("Already active? (F)"=w500, "Target VI reference"=w498, "Error In"=w480, "Abort Button Name (Abort)"=w486) -> ("Error Out"=w501:errorcluster)  [unwired: 15 in]
        }
      }
    }
    frame "Decay:Fit IRF to Logistic Square Gate" {
      # "Fit IRF to Logistic Square Gate"
      n141 = Variant To Data(Variant=w510) -> (data=w509:T28, error out=w519:errorcluster)  [unwired: 2 in]
      n142 = call "Show Animated Busy Icon with Message.vi"("Already active? (F)"=w506, "Message"=w505, "Error In"=w519, "Target VI Refnum"=w507) -> ("Error Out"=w518:errorcluster)  [unwired: 7 in]
      n143 = call "AlliGator Fit to Logistic Square Gated IRF.vi"("error in (no error)"=w518, "Selected Plot Info"=w509) -> ("Error Out"=w504:errorcluster, "Message"=w511:string, "Fitted IRF"=w517:cluster{"t Array":dbl[], "IRF Array":dbl[]})  [unwired: 7 in]
      n144 = call "AlliGator IV ROI Decay.vi"("Get (F)/ Set (T)"=TRUE, "error in (no error)"=w504, "Decay in"=w517, "AlliGator IV DVR in"=w514) -> ("error out"=w512:errorcluster, "AlliGator IV DVR out"=w513:refnum<data-value>)  [unwired: 4 in, 2 out]
      n145 = call "Hide Animated Busy Icon with Message.vi"("Already active? (F)"=w506, "Message"=w505, "Error In"=w512, "Target VI reference"=w507) -> ("Error Out"=w508:errorcluster)  [unwired: 7 in]
    }
    frame "Decay:Fit IRF to Square Gate" {
      # "\"Fit IRF to Square Gate\""
      n146 = Variant To Data(Variant=w542) -> (data=w525:T28, error out=w539:errorcluster)  [unwired: 2 in]
      n147 = call "AlliGator Settings Storage.vi"("AlliGator Settings List"=AlliGator_Settings_List."Fluorescence Decay_Advanced Analysis:Square Pulse Options", "Error In"=w539) -> ("Error Out"=w537:errorcluster, "Variant Data out"=w538:variant)  [unwired: 8 in]
      n148 = call "Show Animated Busy Icon with Message.vi"("Already active? (F)"=w522, "Message"=w532, "Error In"=w539, "Target VI Refnum"=w523) -> ("Error Out"=w541:errorcluster)  [unwired: 7 in]
      n149 = Variant To Data(error in=w537, type=T26 {"Method"=enum."Mode", "# Bins"=100, "Threshold %"=10.0, "Center on Midpoint"=TRUE, "Smoothen Plot"=FALSE} ("Square Pulse Options"), Variant=w538) -> (data=w533:T26, error out=w534:errorcluster)
      n150 = Merge Errors(w541, w534) -> (w535:errorcluster)
      n151 = call "Fit to Square Pulse.vi"("Square Pulse Options"=w533, "error in (no error)"=w535, "Selected Plot Info"=w525) -> ("Error Out"=w521:errorcluster, "Fitted Plot Message"=w526:string, "Fitted Plot"=w529:T46)  [unwired: 6 in]
      n152 = call "AlliGator IV ROI Decay.vi"("Get (F)/ Set (T)"=TRUE, "error in (no error)"=w521, "Decay in"=w529, "AlliGator IV DVR in"=w530) -> ("error out"=w528:errorcluster, "AlliGator IV DVR out"=w531:refnum<data-value>)  [unwired: 4 in, 2 out]
      n153 = call "Hide Animated Busy Icon with Message.vi"("Already active? (F)"=w522, "Error In"=w528, "Target VI reference"=w523) -> ("Error Out"=w524:errorcluster)  [unwired: 8 in]
    }
    frame "Decay:Fit IRF to Tilted Logistic Square Gate" {
      # "\"Fit IRF to Tilted Logistic Square Gate\""
      n154 = Variant To Data(Variant=w559) -> (data=w549:T28, error out=w558:errorcluster)  [unwired: 2 in]
      n155 = call "Show Animated Busy Icon with Message.vi"("Already active? (F)"=w546, "Message"=w556, "Error In"=w558, "Target VI Refnum"=w547) -> ("Error Out"=w557:errorcluster)  [unwired: 7 in]
      n156 = call "AlliGator Fit to Tilted Logistic Square Gated IRF.vi"("error in (no error)"=w557, "Selected Plot Info"=w549) -> ("Error Out"=w545:errorcluster, "Message"=w550:string, "Fitted IRF"=w552:cluster{"t Array":dbl[], "IRF Array":dbl[]})  [unwired: 7 in]
      n157 = call "AlliGator IV ROI Decay.vi"("Get (F)/ Set (T)"=TRUE, "error in (no error)"=w545, "Decay in"=w552, "AlliGator IV DVR in"=w554) -> ("error out"=w553:errorcluster, "AlliGator IV DVR out"=w555:refnum<data-value>)  [unwired: 4 in, 2 out]
      n158 = call "Hide Animated Busy Icon with Message.vi"("Already active? (F)"=w546, "Error In"=w553, "Target VI reference"=w547) -> ("Error Out"=w548:errorcluster)  [unwired: 8 in]
    }
    frame "Decay:Fit to Model IRF" {
      # "\"Fit to Model IRF\""
      n159 = Variant To Data(Variant=w576) -> (data=w566:T28, error out=w575:errorcluster)  [unwired: 2 in]
      n160 = call "Show Animated Busy Icon with Message.vi"("Already active? (F)"=w563, "Message"=w573, "Error In"=w575, "Target VI Refnum"=w564) -> ("Error Out"=w574:errorcluster)  [unwired: 7 in]
      n161 = call "AlliGator Fit to Model IRF.vi"("error in (no error)"=w574, "Selected Plot Info"=w566) -> ("Error Out"=w562:errorcluster, "Message"=w567:string, "Fitted IRF"=w570:cluster{"t Array":dbl[], "IRF Array":dbl[]})  [unwired: 7 in]
      n162 = call "AlliGator IV ROI Decay.vi"("Get (F)/ Set (T)"=TRUE, "error in (no error)"=w562, "Decay in"=w570, "AlliGator IV DVR in"=w572) -> ("error out"=w569:errorcluster, "AlliGator IV DVR out"=w571:refnum<data-value>)  [unwired: 4 in, 2 out]
      n163 = call "Hide Animated Busy Icon with Message.vi"("Already active? (F)"=w563, "Error In"=w569, "Target VI reference"=w564) -> ("Error Out"=w565:errorcluster)  [unwired: 8 in]
    }
    frame "Decay:Fold Decay" {
      # "\"Fold Decay\""
      n164 = Variant To Data(Variant=w599) -> (data=w587:T28, error out=w589:errorcluster)  [unwired: 2 in]
      n165 = call "Show Animated Busy Icon with Message.vi"("Already active? (F)"=w580, "Message"=w579, "Error In"=w589, "Target VI Refnum"=w581) -> ("Error Out"=w583:errorcluster)  [unwired: 7 in]
      n166 = call "AlliGator Get Process Plots Indices.vi"("error in (no error)"=w583, "Selected Plot Info"=w587) -> ("error out"=w588:errorcluster, "Selected Plots"=w585:i32[], "Selected Plot Info (dup)"=w586:T28)  [unwired: 7 in]
      n167 = call "AlliGator Settings Storage.vi"("AlliGator Settings List"=AlliGator_Settings_List."Fluorescence Decay_Decay Pre-Processing:# Folds") -> ("Variant Data out"=w597:variant)  [unwired: 9 in, 1 out]
      n168 = call-poly "Variant to Data.vi"("Variant"=w597) -> ("Value"=w596:u32)  [unwired: 8 in]
      n169 = call "XY Graph Fold Multiple Plots.vi"("error in (no error)"=w588, "# Folds (1)"=w596, "Selected Plots"=w585, "Selected Plot Info"=w586) -> ("error out"=w594:errorcluster, "Folded Plot Message"=w590:string, "Last Folded Plot"=w592:cluster{"t Array":dbl[], "IRF Array":dbl[]}, "Single Plot?"=w584:bool)  [unwired: 4 in]
      n170 = case shown="False" w584 {
        tunnel: w595 -> [w602 w608]
        tunnel: w594 -> [w601 w607]
        tunnel: [w601 w606] -> w593
        tunnel: w592 -> [_ w605]
        tunnel: [w602 w604] -> w591
        frame False {
        }
        frame True {
          n171 = call "AlliGator IV ROI Decay.vi"("Get (F)/ Set (T)"=TRUE, "error in (no error)"=w607, "Decay in"=w605, "AlliGator IV DVR in"=w608) -> ("error out"=w606:errorcluster, "AlliGator IV DVR out"=w604:refnum<data-value>)  [unwired: 4 in, 2 out]
        }
      }
      n172 = call "Hide Animated Busy Icon with Message.vi"("Already active? (F)"=w580, "Error In"=w593, "Target VI reference"=w581) -> ("Error Out"=w582:errorcluster)  [unwired: 8 in]
    }
    frame "Decay:Global Fit of Selected Decays" {
      # "\"Global Fit of Selected Decays\""
      n173 = disable-structure shown="Enabled" {
        disable-tunnel: [w635 _] -> w618
        disable-tunnel: w617 -> [w634 w669]
        disable-tunnel: [w633 w669] -> w616
        disable-tunnel: w615 -> [w632 _]
        disable-tunnel: w614 -> [w627 _]
        disable-tunnel: w613 -> [w626 _]
        disable-tunnel: w612 -> [w624 _]
        disable-tunnel: w611 -> [w623 w670]
        disable-tunnel: [w621 w670] -> w610
        disable-tunnel: [w619 _] -> w609
        frame Disabled {
          n174 = Unbundle By Name(w627) -> ("Registered Events Ctrl Refnums.Decay Graph"=w631:refnum<vi>, "Other AlliGator Ctrl Refnums.Abort Fit"=w625:refnum<vi>)
          n175 = call "AlliGator Check Decay Reference.vi"("AlliGator Internal Variables DVR"=w623) -> ("Error Out"=w620:errorcluster, "Valid Reference?"=w630:bool, "Reference Decay"=w628:cluster{"t Array":dbl[], "I Array":dbl[]}, "AlliGator Internal Variables DVR"=w622:refnum<data-value>, "Message"=w629:string)  [unwired: 3 in, 3 out]
          n176 = case shown="True" w630 {
            tunnel: [w638 w667] -> w619
            tunnel: [w636 w642] -> w635
            tunnel: w634 -> [w639 w658]
            tunnel: [w639 w659] -> w633
            tunnel: w632 -> [_ w640]
            tunnel: w631 -> [_ w653]
            tunnel: w629 -> [w638 _]
            tunnel: w628 -> [_ w652]
            tunnel: w626 -> [_ w651]
            tunnel: w625 -> [_ w650]
            tunnel: w624 -> [_ w649]
            tunnel: [w637 w645] -> w621
            tunnel: w622 -> [w637 w648]
            tunnel: w620 -> [w636 _]
            frame False {
            }
            frame True {
              n177 = call "Show Animated Busy Icon with Message.vi"("Already active? (F)"=w640, "Message"=w649, "Target VI Refnum"=w651) -> ("Error Out"=w665:errorcluster)  [unwired: 8 in]
              n178 = call "AlliGator Global Fit Decays.vi"("IRF"=w652, "error in (no error)"=w665, "Abort Fit"=w650, "Decay Graph"=w653) -> ("Error Out"=w647:errorcluster, "Reduced Chi^2"=w654:dbl, "R^2"=w655:dbl, "Best Fit Parameters"=w666:dbl[], "Fit Output Message"=w667:string, "Aborted?"=w664:bool)  [unwired: 2 in]
              n179 = Build Array (concatenate)(w666, w655, w654) -> (w646:dbl[])
              n180 = call "AlliGator IV Single Fit Parameters.vi"("Get (F)/ Set (T)"=TRUE, "error in (no error)"=w647, "[Single Decay Fit Parameter]"=w646, "AlliGator IV DVR in"=w648) -> ("error out"=w644:errorcluster, "AlliGator IV DVR out"=w645:refnum<data-value>)  [unwired: 5 in, 1 out]
              n181 = Select(t="Fit Aborted!" ("Fit Output Message"), s=w664, f="") -> (s? t:f=w661:string)
              n182 = call "Play Error Sound.vi"("Error In"=w644) -> ("Error Out"=w660:errorcluster)  [unwired: 26 in]
              n183 = call "Hide Animated Busy Icon with Message.vi"("Already active? (F)"=w640, "Message"=w661, "Error In"=w660, "Target VI reference"=w651) -> ("Error Out"=w643:errorcluster)  [unwired: 7 in]
              n184 = flat-sequence {
                tunnel: w642 -> [_]
                frame #0 {
                  n185 = global write "Abort Fit Global.vi" "Abort Fit"(FALSE ("Visible")) -> ()
                }
              }
              n186 = call-poly "AlliGator Add Action(s) to Stack.vi"("Elements Order in Action Stack (Default: 2 BEFORE 1)"=Alligator_Elements_Order_in_Action_Stack."Enqueue 2 BEFORE 1", "Error In"=w643, "Alligator Atomic Action"=T6 {"AlliGator Q Event"=enum."Decay:Post Global Fit Script", "Data"=variant}, "Alligator Queue Element 1"=w658) -> ("Error Out"=w642:errorcluster, "Alligator Queue Element 1 (+ 2)"=w659:T6[])  [unwired: 6 in]
            }
          }
        }
        frame Enabled {
        }
      }
    }
    frame "Decay:Optimal IRF Extraction" {
      # "\"Optimal IRF Extraction\""
      n187 = Variant To Data(Variant=w686) -> (data=w683:T28, error out=w685:errorcluster)  [unwired: 2 in]
      n188 = call "Show Animated Busy Icon with Message.vi"("Already active? (F)"=w673, "Message"=w682, "Error In"=w685, "Target VI Refnum"=w674) -> ("Error Out"=w684:errorcluster)  [unwired: 7 in]
      n189 = call "AlliGator Get Optimal IRF from Decay v2.vi"("error in (no error)"=w684, "Selected Plot Info"=w683) -> ("Error Out"=w672:errorcluster, "Message"=w676:string, "Extracted IRF"=w678:cluster{"t Array":dbl[], "IRF Array":dbl[]})  [unwired: 7 in]
      n190 = call "AlliGator IV ROI Decay.vi"("Get (F)/ Set (T)"=TRUE, "error in (no error)"=w672, "Decay in"=w678, "AlliGator IV DVR in"=w681) -> ("error out"=w679:errorcluster, "AlliGator IV DVR out"=w680:refnum<data-value>)  [unwired: 4 in, 2 out]
      n191 = call "Hide Animated Busy Icon with Message.vi"("Already active? (F)"=w673, "Error In"=w679, "Target VI reference"=w674) -> ("Error Out"=w675:errorcluster)  [unwired: 8 in]
    }
    frame "Decay:Plot Convolution" {
      # "\"Decay:Plot Convolution\""
      n192 = Variant To Data(type=T28 {"Multiplot XY Graph"=refnum, "Mouse Coordinates"={"Horizontal"=0, "Vertical"=0}, "Plot Index"=-1} ("Selected Plot Info"), Variant=w714) -> (data=w706:T28, error out=w702:errorcluster)  [unwired: 1 in]
      n193 = call "Show Animated Busy Icon with Message.vi"("Already active? (F)"=w690, "Message"=w689, "Error In"=w702, "Target VI Refnum"=w691) -> ("Error Out"=w693:errorcluster)  [unwired: 7 in]
      n194 = call "AlliGator IV Reference Decay.vi"("Get (F)/ Set (T)"=FALSE, "Error In"=w693, "AlliGator IV DVR in"=w709) -> ("Error Out"=w703:errorcluster, "Reference Decay"=w704:cluster{"t Array":dbl[], "I Array":dbl[]}, "AlliGator IV DVR out"=w707:refnum<data-value>)  [unwired: 5 in, 1 out]
      n195 = call "AlliGator Get Selected Plots and Reference Decay.vi"("error in (no error)"=w703, "Reference Decay"=w704, "Selected Plot Info"=w706) -> ("error out"=w699:errorcluster, "Valid Reference Decay?"=w700:bool, "Selected Plots"=w697:i32[], "XYGraph"=w701:T24, "Reference Decay"=w698:cluster{"t Array":dbl[], "Value Array":dbl[]})  [unwired: 4 in]
      n196 = for {
        tunnel: [w724] -> w696 mode=indexing if=w716
        tunnel: w701 -> [w722]
        tunnel: w700 -> [w721]
        tunnel: w698 -> [w719]
        tunnel: w697 -> [w718] mode=indexing
        tunnel: w699 -> [w720]
        n197 = call "XY Graph Compute Convolution Product Event.vi"("Reference Decay"=w719, "Error In"=w720, "Valid Reference Decay?"=w721, "Plot at Coordinates"=w718, "Multiplot XY Graph"=w722) -> ("Error Out"=w723:errorcluster, "Message"=w724:string)  [unwired: 4 in, 1 out]
        n198 = Unbundle By Name(w723) -> ("status"=w717:bool)
        n199 = Not(x=w717) -> (.not. x?=w716:bool)
      }
      n200 = call <vilib>:"1D String Array to Delimited String.vi"("delimiter"="\n", "string array"=w696) -> ("delimited string"=w694:string)  [unwired: 9 in]
      n201 = Format Into String(format string="%s: %s", w712, w694) -> (resulting string=w710:string, error out=w711:errorcluster)  [unwired: 2 in]
      n202 = call "Hide Animated Busy Icon with Message.vi"("Already active? (F)"=w690, "Error In"=w711, "Target VI reference"=w691) -> ("Error Out"=w692:errorcluster)  [unwired: 8 in]
    }
    frame "Decay:Post Global Fit Script" {
      # "\"Post Global Fit Script\""
      n203 = Unbundle By Name(w732) -> ("Registered Events Ctrl Refnums.Lifetime Graph"=w733:refnum<vi>)
      n204 = call "AlliGator Post Global Fit Script.vi"("XYGraph in"=w733) -> ("Error Out"=w728:errorcluster, "Q Elements out"=w729:T6[])  [unwired: 9 in]
      n205 = call-poly "AlliGator Add Action(s) to Stack.vi"("Elements Order in Action Stack (Default: 2 BEFORE 1)"=Alligator_Elements_Order_in_Action_Stack."Enqueue 2 BEFORE 1", "Error In"=w728, "Alligator Queue Element 2"=w729, "Alligator Queue Element 1"=w731) -> ("Error Out"=w727:errorcluster, "Alligator Queue Element 1 (+ 2)"=w730:T6[])  [unwired: 6 in]
    }
    frame "Decay:Rebin Plot" {
      # "\"Decay:Rebin Plot\""
      n206 = Variant To Data(Variant=w753) -> (data=w744:T28, error out=w752:errorcluster)  [unwired: 2 in]
      n207 = call "Show Animated Busy Icon with Message.vi"("Already active? (F)"=w736, "Message"=w738, "Error In"=w752, "Target VI Refnum"=w737) -> ("Error Out"=w740:errorcluster)  [unwired: 7 in]
      n208 = call "AlliGator Get Process Plots Indices.vi"("error in (no error)"=w740, "Selected Plot Info"=w744) -> ("error out"=w745:errorcluster, "Selected Plots"=w741:i32[], "Selected Plot Info (dup)"=w743:T28)  [unwired: 7 in]
      n209 = call "XY Graph Rebin Multiple Plots.vi"("error in (no error)"=w745, "Selected Plots"=w741, "Selected Plot Info"=w743) -> ("error out"=w748:errorcluster, "Rebinned Plot Message"=w746:string, "Last Rebinned Plot"=w749:cluster{"t Array":dbl[], "IRF Array":dbl[]}, "Single Plot?"=w742:bool)  [unwired: 5 in]
      n210 = case shown="True" w742 {
        tunnel: [w756 w762] -> w751
        tunnel: w750 -> [w756 w761]
        tunnel: w749 -> [_ w760]
        tunnel: w748 -> [w755 w759]
        tunnel: [w755 w758] -> w747
        frame False {
        }
        frame True {
          n211 = call "AlliGator IV ROI Decay.vi"("Get (F)/ Set (T)"=TRUE, "error in (no error)"=w759, "Decay in"=w760, "AlliGator IV DVR in"=w761) -> ("error out"=w758:errorcluster, "AlliGator IV DVR out"=w762:refnum<data-value>)  [unwired: 4 in, 2 out]
        }
      }
      n212 = call "Hide Animated Busy Icon with Message.vi"("Already active? (F)"=w736, "Error In"=w747, "Target VI reference"=w737) -> ("Error Out"=w739:errorcluster)  [unwired: 8 in]
    }
    frame "Decay:Shift Decay" {
      # "\"Shift Decay\""
      n213 = Variant To Data(Variant=w792) -> (data=w780:T28, error out=w782:errorcluster)  [unwired: 2 in]
      n214 = call "Show Animated Busy Icon with Message.vi"("Already active? (F)"=w765, "Message"=w764, "Error In"=w782, "Target VI Refnum"=w766) -> ("Error Out"=w768:errorcluster)  [unwired: 7 in]
      n215 = call "AlliGator IV Reference Decay.vi"("Get (F)/ Set (T)"=FALSE, "AlliGator IV DVR in"=w788) -> ("Error Out"=w777:errorcluster, "Reference Decay"=w787:cluster{"t Array":dbl[], "I Array":dbl[]}, "AlliGator IV DVR out"=w786:refnum<data-value>)  [unwired: 6 in, 1 out]
      n216 = call "AlliGator Settings Storage.vi"("Get(F)/Set"=FALSE, "AlliGator Settings List"=AlliGator_Settings_List."Fluorescence Decay_Decay Pre-Processing:Decay Shift Parameters") -> ("Error Out"=w775:errorcluster, "Variant Data out"=w776:variant)  [unwired: 8 in]
      n217 = call "AlliGator Get Process Plots Indices.vi"("error in (no error)"=w768, "Selected Plot Info"=w780) -> ("error out"=w781:errorcluster, "Selected Plots"=w770:i32[], "Selected Plot Info (dup)"=w779:T28)  [unwired: 7 in]
      n218 = Variant To Data(error in=w775, Variant=w776) -> (data=w771:T47, error out=w772:errorcluster)  [unwired: 1 in]
      n219 = Merge Errors(w781, w777, w772) -> (w778:errorcluster)
      n220 = call "XY Graph Shift Multiple Plots.vi"("Plot Shift Parameters"=w771, "Reference Decay"=w787, "error in (no error)"=w778, "Selected Plots"=w770, "Selected Plot Info"=w779) -> ("error out"=w783:errorcluster, "Shifted Plot Message"=w784:string, "Last Shifted Plot"=w791:cluster{"t Array":dbl[], "IRF Array":dbl[]}, "Single Plot?"=w769:bool)  [unwired: 3 in]
      n221 = case shown="True" w769 {
        tunnel: w791 -> [_ w801]
        tunnel: [w795 w800] -> w790
        tunnel: [w794 w799] -> w789
        tunnel: w786 -> [w795 w797]
        tunnel: w783 -> [w794 w796]
        frame False {
        }
        frame True {
          n222 = call "AlliGator IV ROI Decay.vi"("Get (F)/ Set (T)"=TRUE, "error in (no error)"=w796, "Decay in"=w801, "AlliGator IV DVR in"=w797) -> ("error out"=w799:errorcluster, "AlliGator IV DVR out"=w800:refnum<data-value>)  [unwired: 4 in, 2 out]
        }
      }
      n223 = call "Hide Animated Busy Icon with Message.vi"("Already active? (F)"=w765, "Error In"=w789, "Target VI reference"=w766) -> ("Error Out"=w767:errorcluster)  [unwired: 8 in]
    }
    frame "Decay:Show Reference Decay/IRF" {
      # "\"Show Reference Decay/IRF\""
      n224 = Unbundle By Name(w805) -> ("Registered Events Ctrl Refnums.Decay Graph"=w809:refnum<vi>)
      n225 = call "AlliGator Check Decay Reference.vi"("AlliGator Internal Variables DVR"=w804) -> ("Error Out"=w803:errorcluster, "Valid Reference?"=w806:bool, "Reference Decay"=w808:cluster{"t Array":dbl[], "I Array":dbl[]}, "AlliGator Internal Variables DVR"=w802:refnum<data-value>, "Reference Decay Plot Name"=w807:string)  [unwired: 3 in, 3 out]
      n226 = case shown="True" w806 {
        tunnel: w807 -> [_ w818]
        tunnel: w808 -> [_ w819]
        tunnel: w809 -> [_ w820]
        tunnel: [w813 w816] -> w810
        tunnel: w803 -> [w813 w815]
        frame False {
          n227 = call "Play Error Sound.vi"() -> ()  [unwired: 27 in, 1 out]
          n228 = One Button Dialog(message="No Valid Reference Decay/IRF !") -> ()  [unwired: 1 in, 1 out]
        }
        frame True {
          n229 = call-poly "XY Graph Add Plot(s) with Name(s).vi"("XYGraph Ref in"=w820, "Plot Interpolation (Previous Plot's Style)"=LabVIEW_Plot_Interpolation."Line (-)", "Plot"=w819, "Plot Name (\"Plot\")"=w818, "error in (no error)"=w815) -> ("error out"=w816:errorcluster)  [unwired: 7 in, 3 out]
        }
      }
    }
    frame "Decay:Smoothen Plot Tail" {
      # "\"Smoothen Plot\""
      n230 = Variant To Data(Variant=w844) -> (data=w831:T28, error out=w843:errorcluster)  [unwired: 2 in]
      n231 = call "Show Animated Busy Icon with Message.vi"("Already active? (F)"=w822, "Message"=w824, "Error In"=w843, "Target VI Refnum"=w823) -> ("Error Out"=w826:errorcluster)  [unwired: 7 in]
      n232 = call "AlliGator Settings Storage.vi"("AlliGator Settings List"=AlliGator_Settings_List."Fluorescence Decay_Decay Pre-Processing:Smoothing Parameter") -> ("Variant Data out"=w841:variant)  [unwired: 9 in, 1 out]
      n233 = call-poly "Variant to Data.vi"("Variant"=w841) -> ("Value"=w840:dbl)  [unwired: 8 in]
      n234 = call "AlliGator Get Process Plots Indices.vi"("error in (no error)"=w826, "Selected Plot Info"=w831) -> ("error out"=w832:errorcluster, "Selected Plots"=w829:i32[], "Selected Plot Info (dup)"=w830:T28)  [unwired: 7 in]
      n235 = expression code="1-10**(-x)"(w840) -> (w833:dbl)
      n236 = call "XY Graph Smoothen Multiple Plots (Cubic Spline).vi"("balance parameter (-1: auto)"=w833, "error in (no error)"=w832, "Tail only (F)"=TRUE, "Selected Plots"=w829, "Selected Plot Info"=w830) -> ("error out"=w835:errorcluster, "Smoothened Plot Message"=w834:string, "Last Smoothened Plot"=w837:cluster{"t Array":dbl[], "IRF Array":dbl[]}, "Single Plot?"=w827:bool)  [unwired: 3 in]
      n237 = case shown="True" w827 {
        tunnel: w839 -> [w847 w853]
        tunnel: [w847 w852] -> w838
        tunnel: w837 -> [_ w851]
        tunnel: [w846 w850] -> w836
        tunnel: w835 -> [w846 w849]
        frame False {
        }
        frame True {
          n238 = call "AlliGator IV ROI Decay.vi"("Get (F)/ Set (T)"=TRUE, "error in (no error)"=w849, "Decay in"=w851, "AlliGator IV DVR in"=w853) -> ("error out"=w850:errorcluster, "AlliGator IV DVR out"=w852:refnum<data-value>)  [unwired: 4 in, 2 out]
        }
      }
      n239 = call "Hide Animated Busy Icon with Message.vi"("Already active? (F)"=w822, "Error In"=w836, "Target VI reference"=w823) -> ("Error Out"=w825:errorcluster)  [unwired: 8 in]
    }
    frame "Decay:Smoothen Plot" {
      # "\"Smoothen Plot\""
      n240 = Variant To Data(Variant=w877) -> (data=w864:T28, error out=w876:errorcluster)  [unwired: 2 in]
      n241 = call "Show Animated Busy Icon with Message.vi"("Already active? (F)"=w856, "Message"=w855, "Error In"=w876, "Target VI Refnum"=w857) -> ("Error Out"=w859:errorcluster)  [unwired: 7 in]
      n242 = call "AlliGator Settings Storage.vi"("AlliGator Settings List"=AlliGator_Settings_List."Fluorescence Decay_Decay Pre-Processing:Smoothing Parameter") -> ("Variant Data out"=w874:variant)  [unwired: 9 in, 1 out]
      n243 = call-poly "Variant to Data.vi"("Variant"=w874) -> ("Value"=w873:dbl)  [unwired: 8 in]
      n244 = call "AlliGator Get Process Plots Indices.vi"("error in (no error)"=w859, "Selected Plot Info"=w864) -> ("error out"=w865:errorcluster, "Selected Plots"=w862:i32[], "Selected Plot Info (dup)"=w863:T28)  [unwired: 7 in]
      n245 = expression code="1-10**(-x)"(w873) -> (w866:dbl)
      n246 = call "XY Graph Smoothen Multiple Plots (Cubic Spline).vi"("balance parameter (-1: auto)"=w866, "error in (no error)"=w865, "Tail only (F)"=FALSE, "Selected Plots"=w862, "Selected Plot Info"=w863) -> ("error out"=w868:errorcluster, "Smoothened Plot Message"=w867:string, "Last Smoothened Plot"=w870:cluster{"t Array":dbl[], "IRF Array":dbl[]}, "Single Plot?"=w860:bool)  [unwired: 3 in]
      n247 = case shown="True" w860 {
        tunnel: w872 -> [w880 w886]
        tunnel: [w880 w885] -> w871
        tunnel: w870 -> [_ w884]
        tunnel: [w879 w883] -> w869
        tunnel: w868 -> [w879 w882]
        frame False {
        }
        frame True {
          n248 = call "AlliGator IV ROI Decay.vi"("Get (F)/ Set (T)"=TRUE, "error in (no error)"=w882, "Decay in"=w884, "AlliGator IV DVR in"=w886) -> ("error out"=w883:errorcluster, "AlliGator IV DVR out"=w885:refnum<data-value>)  [unwired: 4 in, 2 out]
        }
      }
      n249 = call "Hide Animated Busy Icon with Message.vi"("Already active? (F)"=w856, "Error In"=w869, "Target VI reference"=w857) -> ("Error Out"=w858:errorcluster)  [unwired: 8 in]
    }
    frame "Decay:Store Cursor-defined Head & Tail Fractions" {
      # "\"Store Cursor-defined Head & Tail Fractions\""
      n250 = Variant To Data(Variant=w891) -> (data=w887:T28, error out=w890:errorcluster)  [unwired: 2 in]
      n251 = call "AlliGator Store Cursor-defined Head & Tail Fractions.vi"("error in (no error)"=w890, "Selected Plot Info"=w887) -> ("Error Out"=w892:errorcluster, "Message"=w888:string)  [unwired: 8 in]
    }
    frame "Decay:Straighten Decay" {
      # "\"Straighten Decay\""
      n252 = Variant To Data(Variant=w913) -> (data=w904:T28, error out=w912:errorcluster)  [unwired: 2 in]
      n253 = call "Show Animated Busy Icon with Message.vi"("Already active? (F)"=w896, "Message"=w898, "Error In"=w912, "Target VI Refnum"=w897) -> ("Error Out"=w900:errorcluster)  [unwired: 7 in]
      n254 = call "AlliGator Get Process Plots Indices.vi"("error in (no error)"=w900, "Selected Plot Info"=w904) -> ("error out"=w905:errorcluster, "Selected Plots"=w902:i32[], "Selected Plot Info (dup)"=w903:T28)  [unwired: 7 in]
      n255 = call "XY Graph Straighten Multiple Decays.vi"("error in (no error)"=w905, "Selected Plots"=w902, "Selected Plot Info"=w903) -> ("error out"=w908:errorcluster, "Straightened Plot Message"=w906:string, "Last Straightened Plot"=w909:cluster{"t Array":dbl[], "IRF Array":dbl[]}, "Single Plot?"=w901:bool)  [unwired: 5 in]
      n256 = case shown="True" w901 {
        tunnel: w911 -> [w916 w922]
        tunnel: [w916 w921] -> w910
        tunnel: w909 -> [_ w920]
        tunnel: w908 -> [w915 w919]
        tunnel: [w915 w918] -> w907
        frame False {
        }
        frame True {
          n257 = call "AlliGator IV ROI Decay.vi"("Get (F)/ Set (T)"=TRUE, "error in (no error)"=w919, "Decay in"=w920, "AlliGator IV DVR in"=w922) -> ("error out"=w918:errorcluster, "AlliGator IV DVR out"=w921:refnum<data-value>)  [unwired: 4 in, 2 out]
        }
      }
      n258 = call "Hide Animated Busy Icon with Message.vi"("Already active? (F)"=w896, "Error In"=w907, "Target VI reference"=w897) -> ("Error Out"=w899:errorcluster)  [unwired: 8 in]
    }
    frame "Decay:Threshold IRF" {
      # "\"Threshold IRF\""
      n259 = Variant To Data(Variant=w938) -> (data=w929:T28, error out=w937:errorcluster)  [unwired: 2 in]
      n260 = call "Show Animated Busy Icon with Message.vi"("Already active? (F)"=w925, "Message"=w924, "Error In"=w937, "Target VI Refnum"=w926) -> ("Error Out"=w928:errorcluster)  [unwired: 7 in]
      n261 = call "AlliGator Thresholded IRF.vi"("error in (no error)"=w928, "Selected Plot Info"=w929) -> ("Error Out"=w933:errorcluster, "Message"=w930:string, "Thresholded IRF"=w934:cluster{"t Array":dbl[], "IRF Array":dbl[]})  [unwired: 7 in]
      n262 = call "AlliGator IV ROI Decay.vi"("Get (F)/ Set (T)"=TRUE, "error in (no error)"=w933, "Decay in"=w934, "AlliGator IV DVR in"=w936) -> ("error out"=w932:errorcluster, "AlliGator IV DVR out"=w935:refnum<data-value>)  [unwired: 4 in, 2 out]
      n263 = call "Hide Animated Busy Icon with Message.vi"("Already active? (F)"=w925, "Error In"=w932, "Target VI reference"=w926) -> ("Error Out"=w927:errorcluster)  [unwired: 8 in]
    }
    frame "Decay:Use as Reference Decay" {
      w945 = TRUE ("ON/OFF")
      # "\"Use as Reference Decay\""
      n264 = Variant To Data(Variant=w963) -> (data=w950:T28, error out=w949:errorcluster)  [unwired: 2 in]
      n265 = Unbundle By Name(w958) -> ("Other AlliGator Ctrl Refnums.State Indicators"=w959:refnum<vi>)
      n266 = call "Show Animated Busy Icon with Message.vi"("Already active? (F)"=w940, "Message"=w942, "Error In"=w949, "Target VI Refnum"=w941) -> ("Error Out"=w944:errorcluster)  [unwired: 7 in]
      n267 = call "XY Graph Get Selected Plot.vi"("error in (no error)"=w944, "Selected Plot Info"=w950) -> ("error out"=w948:errorcluster, "Plot Name"=w947:string, "Plot"=w946:T35)  [unwired: 4 in, 3 out]
      n268 = call "AlliGator Get-Set State Indicators.vi"("State Indicators Refnum"=w959, "AlliGator State Indicators List"=AlliGator_State_Indicators_List."Reference/IRF Defined", "Error In"=w948, "ON/OFF"=w945, "Set (T)/Get"=w945) -> ("Error Out"=w953:errorcluster)  [unwired: 8 in, 2 out]
      n269 = call "AlliGator IV Reference Decay.vi"("Get (F)/ Set (T)"=TRUE, "Error In"=w953, "Reference Decay Plot Name"=w947, "Reference Decay"=w946, "AlliGator IV DVR in"=w956) -> ("Error Out"=w952:errorcluster, "AlliGator IV DVR out"=w957:refnum<data-value>)  [unwired: 3 in, 2 out]
      n270 = Format Into String(format string="%s: %s", error in=w952, w961, w947) -> (resulting string=w951:string, error out=w960:errorcluster)  [unwired: 1 in]
      n271 = call "Hide Animated Busy Icon with Message.vi"("Already active? (F)"=w940, "Error In"=w960, "Target VI reference"=w941) -> ("Error Out"=w943:errorcluster)  [unwired: 8 in]
    }
    frame Default {
      # "\"---- Decays ----\""
    }
  }
  "AlliGator IV DVR out" <- w18
  "error out" <- w1
  "AlliGator Q Elements out" <- w11
  "Script off" <- w8
  n272 = call "Get Current Message Text Format.vi"("Text Format"=w3) -> ("Error Out"=w2:errorcluster, "Message Formatting"=w4:T2)  [unwired: 8 in]
  n273 = call "AlliGator Package Notebook Messages.vi"("Error In"=w2, "Message Formatting"=w4, "Message"=w6, "AlliGator Q Event in"="AlliGator Q Event in") -> ("[Notebook Message]"=→"[Notebook Message]":T1[])  [unwired: 6 in, 1 out]
